vi "luch 2 in 1 - 2v.vi"() -> ()   [LabVIEW 2016]
panel:
  in  "Setup 2":bool
  in  "IBP":bool
  in  "Setup":bool
  in  "Values start":T1=5 items=["External rising edge"=1, "Single shot internal rising edge"=3, "Single shot"=5]
  in  "DZ2K1W":bool
  in  "BZ2K1W":bool
  in  "BZ1K1W":bool
  in  "DZ1K1W":bool
  out "I F0-ethernet 1":string
  in  "F0-ethernet 1":bool
  out "F0-e 3":bool
  out "I: GF":string
  out "GF":bool
  in  "Delay D (0 s)":ext=100.0
  in  "GF":bool
  out "I: FI":string
  out "FI":bool
  in  "Delay C (0 s)":ext=100.0
  in  "FI":bool
  in  "F-R VISAR1":bool
  in  "Delay A (0 s)":ext=100.0
  out "F-R VISAR 1":bool
  out "I: F-R VISAR 1":string
  out "F-R VISAR 2":bool
  out "I: F-R VISAR 2":string
  in  "F-R VISAR2":bool
  in  "Delay B (0 s)":ext=100.0
  in  "WebBrowser":refnum<k7>(container)
  out "Time Stamp":T2
  in  "stop":T3
  out "VISA resource name out":string
  out "I: DZ2K1W":string
  out "DZ2K1W":bool
  out "I: BZ2K1W":string
  out "BZ2K1W":bool
  out "I: BZ1K1W":string
  out "BZ1K1W":bool
  out "I: DZ1K1W":string
  out "DZ1K1W":bool
  out "I: F0-ethernet 5":string
  in  "F0-ethernet 5":bool
  out "F0-e 5":bool
  in  "GF":bool
  in  "FI":bool
  in  "F-R VISAR 4":bool
  in  "F-R VISAR 3":bool
  out "I: BZ1K2W":string
  out "BZ1K2W":bool
  out "I: DZ1K2W":string
  out "DZ1K2W":bool
  out "I: F0-ethernet 4":string
  in  "F0-ethernet 4":bool
  out "F0-e 4":bool
  out "I: BZ2K2W":string
  out "I: DZ2K2W":string
  out "DZ2K2W":bool
  out "BZ2K2W":bool
  in  "BK3":bool
  in  "BK 2":bool
  in  "BK1":bool
  in  "Kamera Y":bool
  out "mod 02":string
  out "mod 01":string
  out "I F0-ethernet 3":string
  in  "F0-ethernet 3":bool
  out "F0-e 1":bool
  out "I: PZS 2 DOP":string
  out "I: PZS 1 DOP":string
  in  "PZS 2 DOP":bool
  in  "PZS 1 DOP":bool
  out "PZS 2 DOP":bool
  out "PZS 1 DOP":bool
  in  "BZ1K2W":bool
  in  "DZ1K2W":bool
  in  "BZ2K2W":bool
  in  "DZ2K2W":bool
  out "I: BK3":string
  out "BK3":bool
  in  "Delay H (0 s)":ext=100.0
  in  "BK3":bool
  in  "Delay G (0 s)":ext=100.0
  in  "BK2":bool
  out "I: BK2":string
  out "BK2":bool
  in  "Delay F (0 s)":ext=100.0
  in  "BK1":bool
  out "I: BK1":string
  out "BK1":bool
  out "I F0-ethernet 2":string
  in  "Delay E (0 s)":ext=100.0
  in  "Kamera Y":bool
  out "I: Kamera Y":string
  out "Kamera Y":bool
  in  "F0-ethernet 2":bool
  out "F0-e 2":bool
  out "error out 2":errorcluster
  out "I 0_3":string
  in  "rele 0_6":bool
  out "modul 03":string
  out "0_3":bool
  out "error out":errorcluster
  # "Ток(A)"
  # "FO-ETHERNET №2"
  # "Гармоника 2"
  # "Ток(A)"
  # "Камеру У"
  # "Камера Б1"
  # "Ток(A)"
  # "Ток(A)"
  # "FO-ETHERNET №4"
  # "1 канал Дальняя Зона"
  # "2 канал Дальняя Зона"
  # "Ток(A)"
  # "Ток(A)"
  # "Задержка E (100~1099ns)"
  # "Задержка F (100~1099ns)"
  # "1 канал Ближняя Зона"
  # "2 канал Ближняя Зона"
  # "Ток(A)"
  # "Ток(A)"
  # "Камера Б2"
  # "Камера Б3"
  # "Ток(A)"
  # "Ток(A)"
  # "Ток(A)"
  # "Гармоника 1"
  # "FO-ETHERNET №5"
  # "1 канал Дальняя Зона"
  # "2 канал Дальняя Зона"
  # "Ток(A)"
  # "Ток(A)"
  # "Ток(A)"
  # "FO-ETHERNET №3"
  # "2 канал Ближняя Зона"
  # "1 канал Ближняя Зона"
  # "Ток (A)"
  # "Ток(A)"
  # "Ток(A)"
  # "ПЗС №1"
  # "Ток(A)"
  # "ПЗС №2"
  # "ИСТОЧНИК БЕСПИРИБОЙНОГО ПИТАНИЯ"
  # "Ток(A)"
  # "FO-ETHERNET №1"
  # "VISAR №2"
  # "VISAR №1"
  # "Ток(A)"
  # "Ток(A)"
  # "Задержка А (100~1099ns)"
  # "Задержка B (100~1099ns)"
  # "Форма имульса"
  # "Глубокий фронт"
  # "Ток(A)"
  # "Ток(A)"
  # "Задержка С (100~1099ns)"
  # "Задержка D (100~1099ns)"
  # "Задержка H (100~1099ns)"
  # "Задержка G (100~1099ns)"
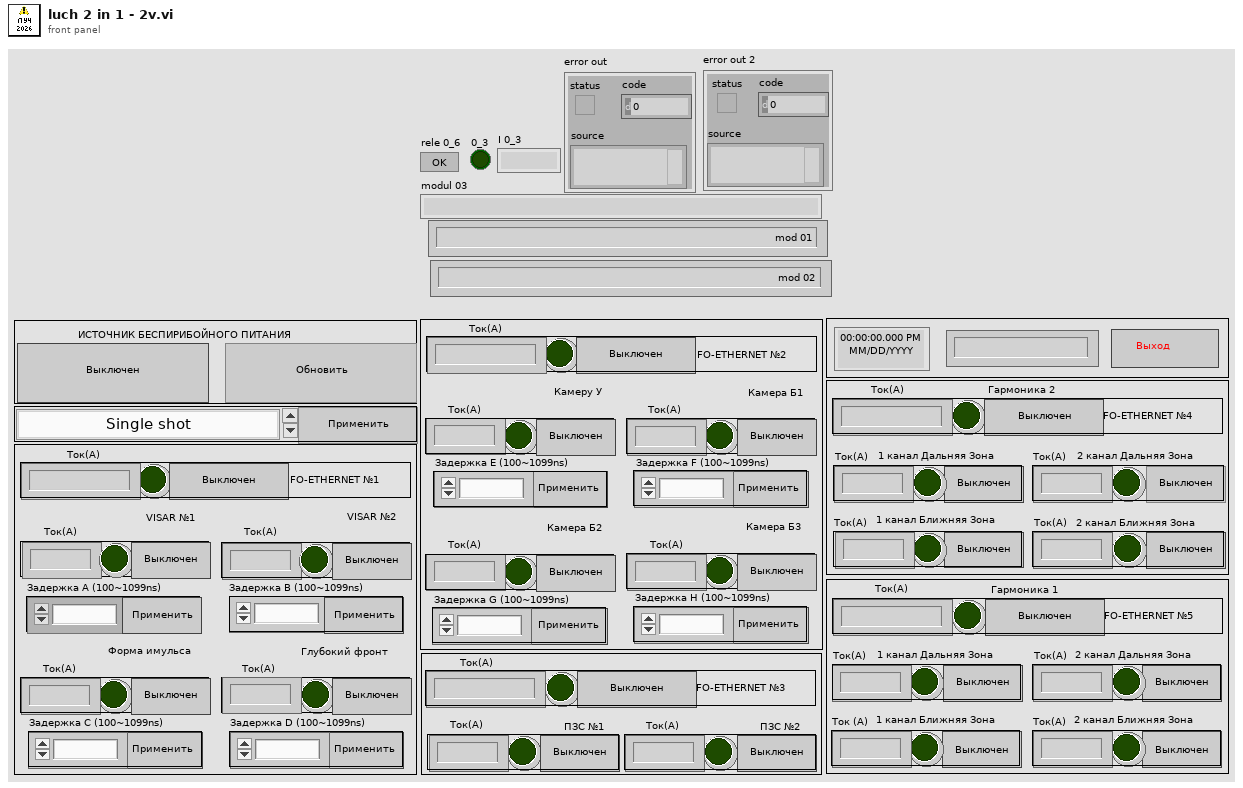
[diagram p1: front panel]
types:
  T1 = typedef "Control 2.ctl" = u16
  T2 = typedef "Control 4.ctl" = timestamp
  T3 = typedef "Control 1.ctl" = bool
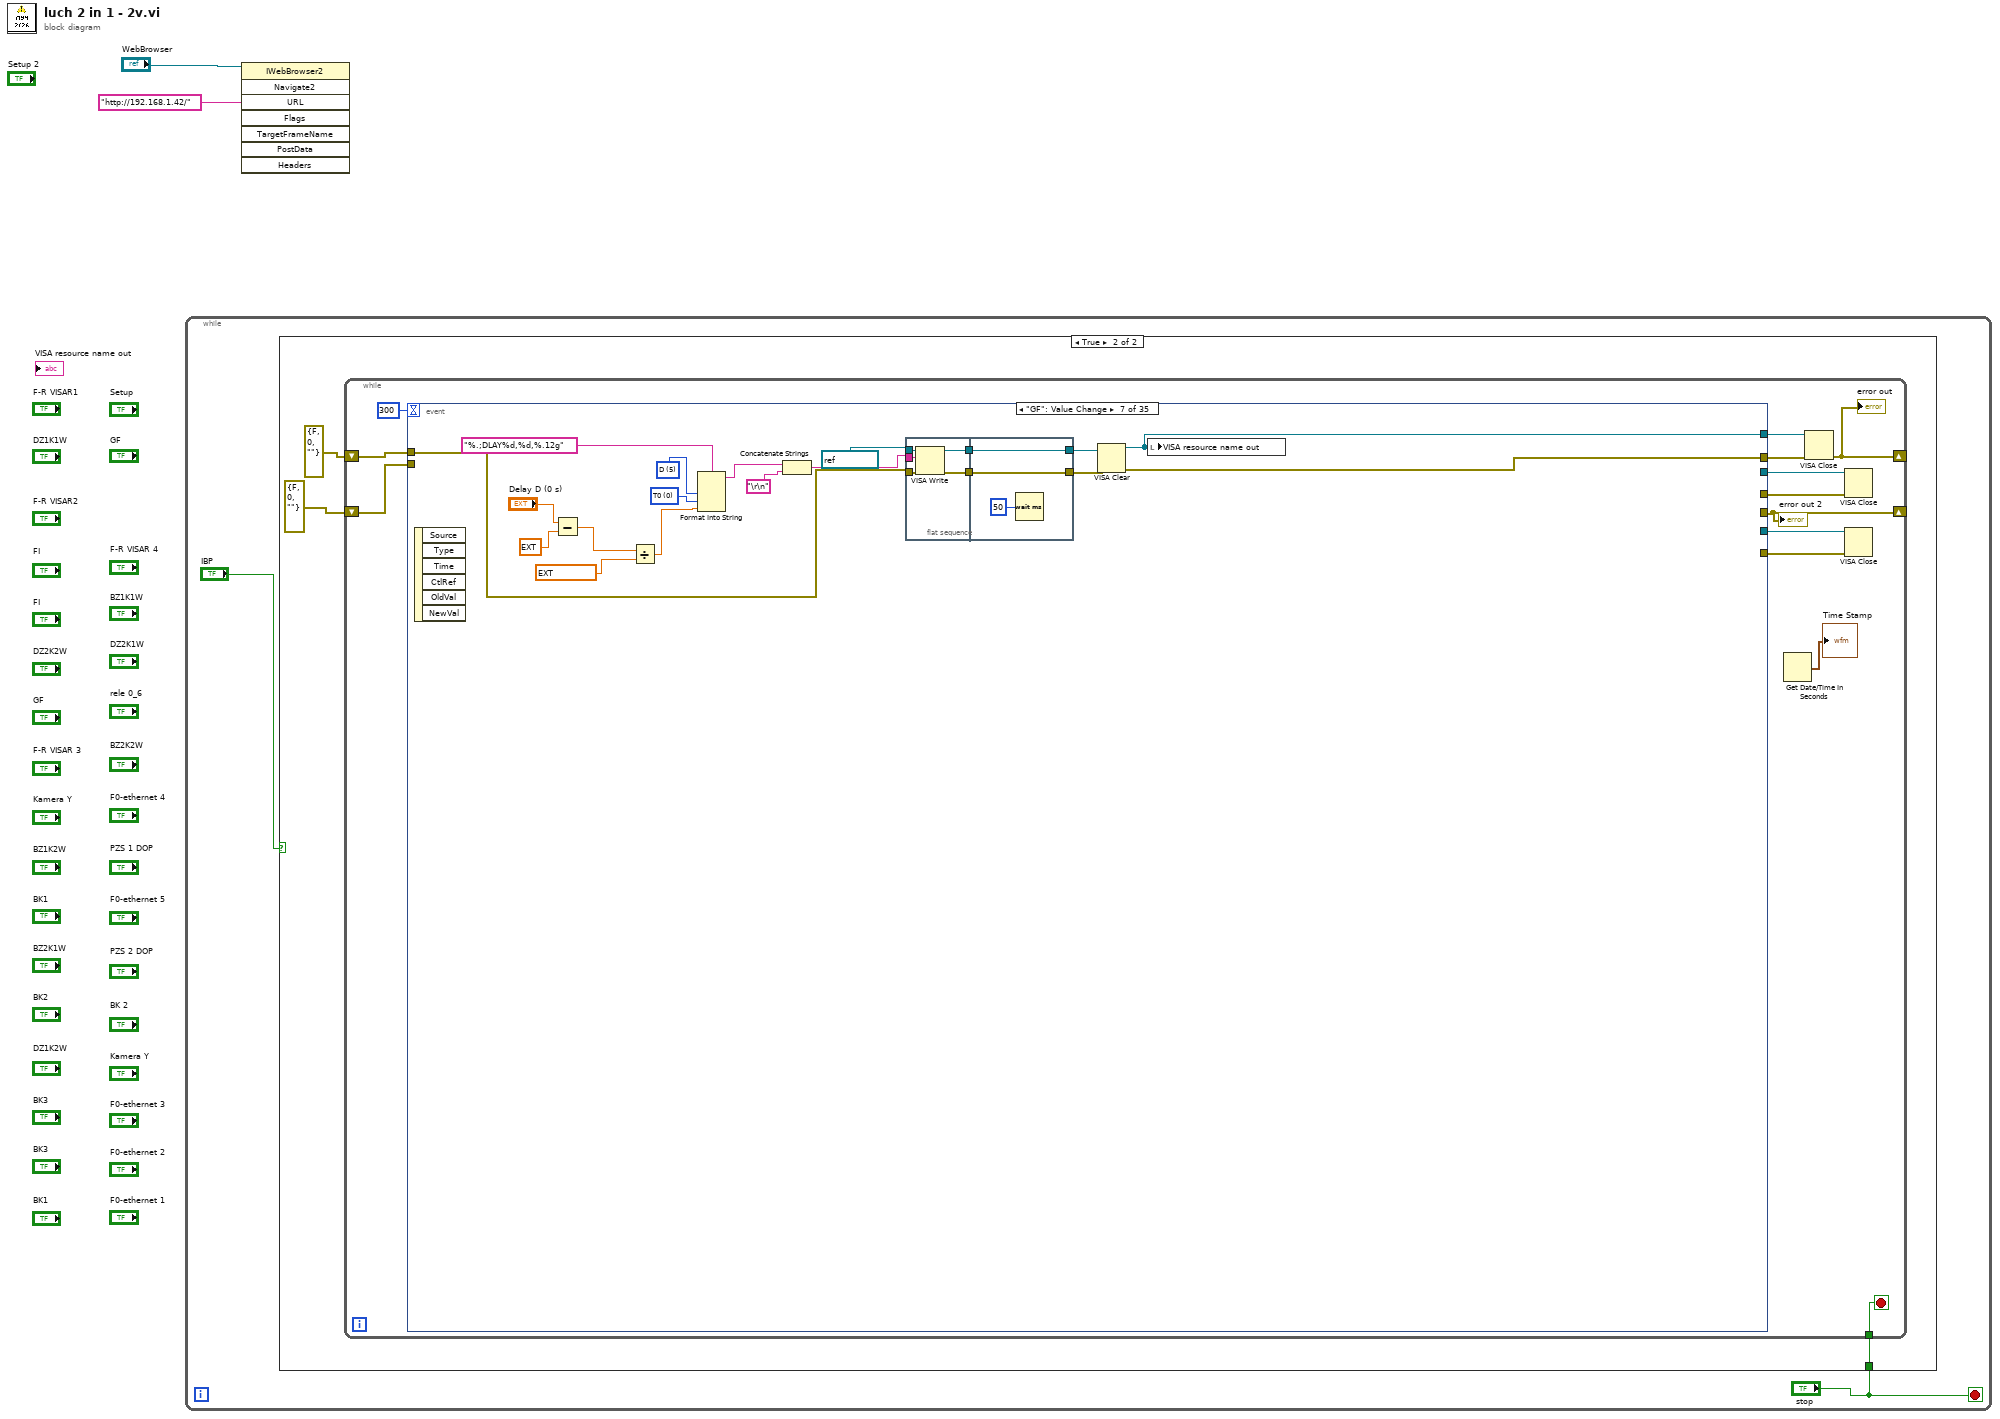
[diagram p0: block diagram]
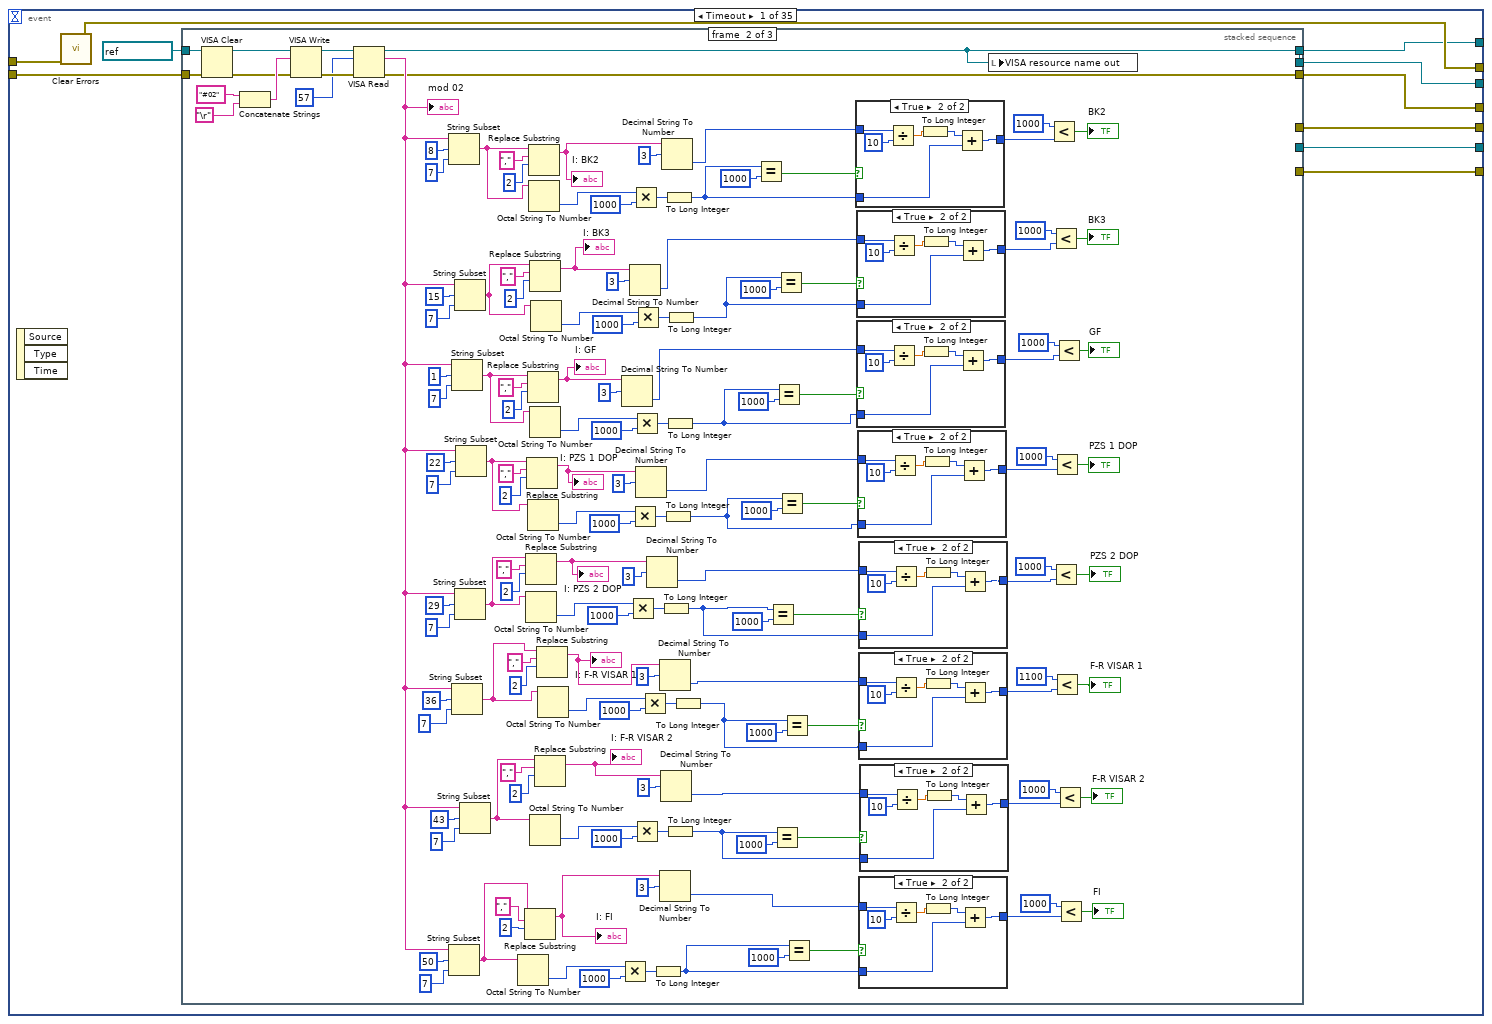
[diagram p3: hidden frame]
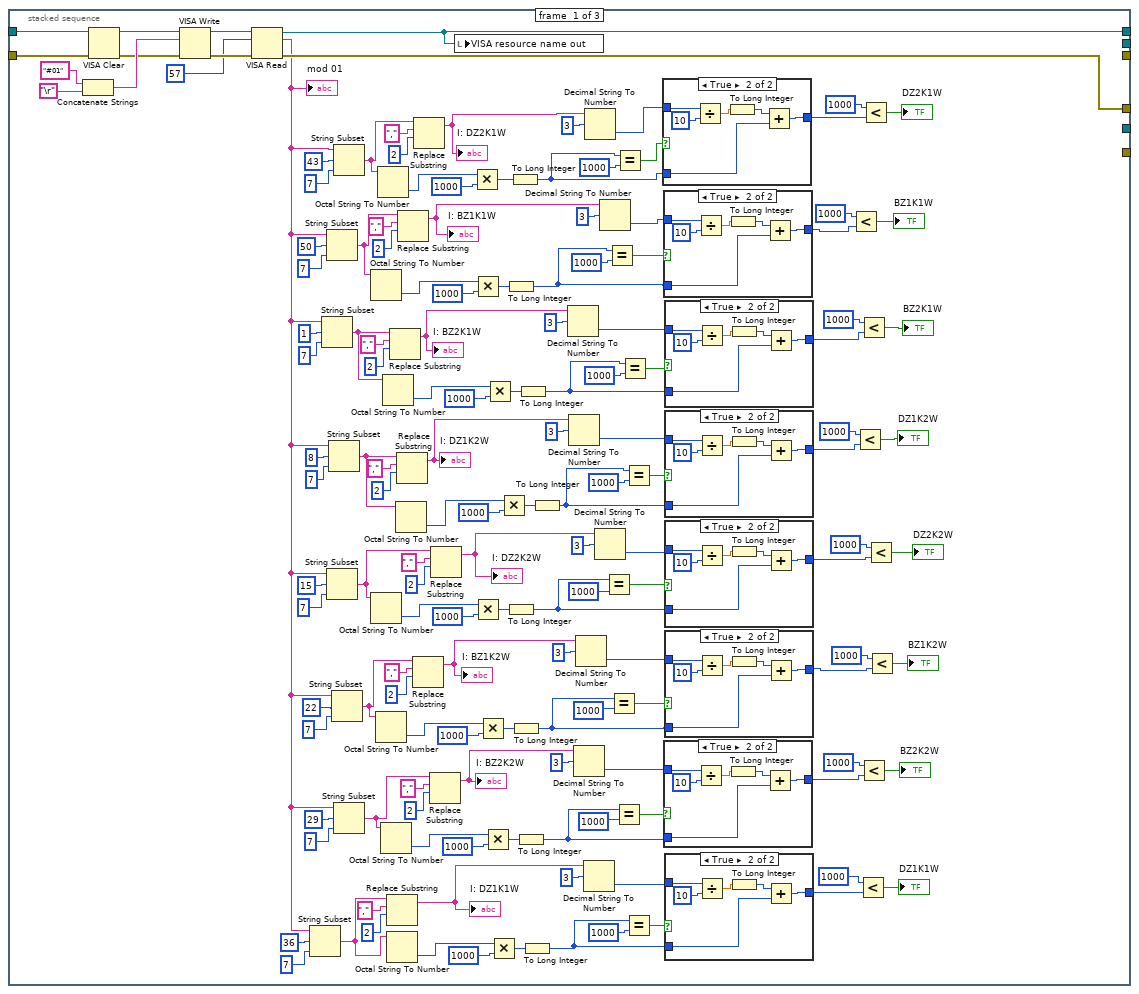
[diagram p4: hidden frame]
diagram:
  n1 = while {
    stop <- "stop" stop-if-true
    n2 = case shown="True" "IBP" {
      tunnel: "stop" -> [_ w5]
      frame False {
      }
      frame True {
        n3 = while {
          shift-right: [w18] -> _
          shift-left: errorcluster {"status"=FALSE, "code"=0, "source"=""} ("error out") -> [w20]
          shift-right: [w11] -> _
          shift-left: errorcluster {"status"=FALSE, "code"=0, "source"=""} ("error out") -> [w19]
          tunnel: w5 -> [w8]
          stop <- w8 stop-if-true
          n4 = event shown="[6] \"GF\": Value Change" {
            selector: _ -> [_ _ _ _ _ _ _ _ _ _ _ _ _ _ _ _ _ _ _ _ _ _ _ _ _ _ _ _ _ _ _ _ _ _ _]
            dyn-events: _ -> [_ _ _ _ _ _ _ _ _ _ _ _ _ _ _ _ _ _ _ _ _ _ _ _ _ _ _ _ _ _ _ _ _ _ _]
            timeout: 300 -> [_ _ _ _ _ _ _ _ _ _ _ _ _ _ _ _ _ _ _ _ _ _ _ _ _ _ _ _ _ _ _ _ _ _ _]
            tunnel: [w29 w647 w650 w720 w747 w775 w801 w828 w854 w882 w909 _ _ _ _ _ _ _ _ _ _ _ _ _ _ _ _ _ _ _ _ _ _ _ _] -> w12
            tunnel: w20 -> [w30 w648 w652 w723 w750 w777 w804 w831 w858 w885 w912 _ _ _ _ _ _ _ _ _ _ _ _ _ _ _ _ _ _ _ _ _ _ _ _]
            tunnel: w19 -> [w27 w644 _ _ _ _ _ _ _ _ _ w934 w962 w995 w1026 w1057 w1088 w1119 w1150 w1181 w1213 w1243 w1274 w1305 w1336 w1367 w1399 w1429 w1460 w1491 w1522 w1553 w1584 w1615 w1646]
            tunnel: [w26 w643 _ _ _ _ _ _ _ _ _ w930 w961 w992 w1023 w1055 w1085 w1117 w1147 w1178 w1209 w1240 w1271 w1302 w1333 w1364 w1395 w1426 w1457 w1488 w1519 w1550 w1581 w1612 w1643] -> w11
            tunnel: [w25 _ w649 w716 w743 w770 w797 w824 w851 w878 w905 w927 w958 w989 w1020 w1051 w1082 w1113 w1144 w1175 w1206 w1237 w1268 w1299 w1330 w1361 w1392 w1423 w1454 w1485 w1516 w1547 w1578 w1609 w1640] -> w17
            tunnel: [w24 _ _ _ _ _ _ _ _ _ _ _ _ _ _ _ _ _ _ _ _ _ _ _ _ _ _ _ _ _ _ _ _ _ _] -> w16
            tunnel: [w23 _ _ _ _ _ _ _ _ _ _ _ _ _ _ _ _ _ _ _ _ _ _ _ _ _ _ _ _ _ _ _ _ _ _] -> w15
            tunnel: [w22 _ _ _ _ _ _ _ _ _ _ _ _ _ _ _ _ _ _ _ _ _ _ _ _ _ _ _ _ _ _ _ _ _ _] -> w14
            tunnel: [w21 _ _ _ _ _ _ _ _ _ _ _ _ _ _ _ _ _ _ _ _ _ _ _ _ _ _ _ _ _ _ _ _ _ _] -> w13
            event Timeout {
              n5 = event-data() -> ()  [unwired: 1 in, 3 out]
              n6 = call <vilib>:"Clear Errors.vi"("error in (no error)"=w30) -> ("error out"=w29:errorcluster)  [unwired: 5 in, 1 out]
              n7 = stacked-sequence {
                tunnel: refnum<visa-resource-name> "Adam" ("VISA resource name") -> [w107 w311 w535]
                tunnel: [w141 _ _] -> w26
                tunnel: w27 -> [w106 w313 w532]
                tunnel: [w103 _ _] -> w25
                tunnel: [_ w309 _] -> w24
                tunnel: [_ w308 _] -> w23
                tunnel: [_ _ w515] -> w22
                tunnel: [_ _ w514] -> w21
                frame #0 {
                  n8 = Concatenate Strings("#01" ("string"), "\r") -> (w179:string)
                  n9 = VISA Clear(VISA resource name=w107, error in (no error)=w106) -> (VISA resource name out=w104:refnum<visa-resource-name>, error out=w105:errorcluster)
                  n10 = VISA Write(VISA resource name=w104, write buffer=w179, error in (no error)=w105) -> (VISA resource name out=w144:refnum<visa-resource-name>, error out=w143:errorcluster)  [unwired: 1 out]
                  n11 = VISA Read(VISA resource name=w144, byte count=u32 57, error in (no error)=w143) -> (VISA resource name out=w103:refnum<visa-resource-name>, read buffer=w124:string, error out=w141:errorcluster)  [unwired: 1 out]
                  "mod 01" <- w124
                  n12 = String Subset(string=w124, offset (0)=36, length (rest)=7 ("length (rest)")) -> (substring=w98:string)
                  n13 = String Subset(string=w124, offset (0)=1, length (rest)=7 ("length (rest)")) -> (substring=w53:string)
                  n14 = String Subset(string=w124, offset (0)=50, length (rest)=7 ("length (rest)")) -> (substring=w43:string)
                  n15 = String Subset(string=w124, offset (0)=15, length (rest)=7 ("length (rest)")) -> (substring=w71:string)
                  n16 = String Subset(string=w124, offset (0)=8, length (rest)=7 ("length (rest)")) -> (substring=w58:string)
                  n17 = String Subset(string=w124, offset (0)=22, length (rest)=7 ("length (rest)")) -> (substring=w76:string)
                  n18 = String Subset(string=w124, offset (0)=43, length (rest)=7 ("length (rest)")) -> (substring=w34:string)
                  n19 = String Subset(string=w124, offset (0)=29, length (rest)=7 ("length (rest)")) -> (substring=w88:string)
                  n20 = Octal String To Number(4:w43) -> (0:w47:u32)  [unwired: 2 in, 1 out]
                  n21 = Octal String To Number(4:w71) -> (0:w75:u32)  [unwired: 2 in, 1 out]
                  n22 = Octal String To Number(4:w76) -> (0:w82:u32)  [unwired: 2 in, 1 out]
                  n23 = Octal String To Number(4:w34) -> (0:w38:u32)  [unwired: 2 in, 1 out]
                  n24 = Octal String To Number(4:w88) -> (0:w91:u32)  [unwired: 2 in, 1 out]
                  n25 = Octal String To Number(4:w53) -> (0:w57:u32)  [unwired: 2 in, 1 out]
                  n26 = Replace Substring(3:2 ("offset (0)"), 4:"," ("substring (\"\")"), 5:w98) -> (1:w112:string)  [unwired: 1 in, 1 out]
                  "I: DZ1K1W" <- w112
                  n27 = Octal String To Number(4:w98) -> (0:w102:u32)  [unwired: 2 in, 1 out]
                  n28 = Replace Substring(3:2 ("offset (0)"), 4:"," ("substring (\"\")"), 5:w53) -> (1:w123:string)  [unwired: 1 in, 1 out]
                  "I: BZ2K1W" <- w123
                  n29 = Octal String To Number(4:w58) -> (0:w66:u32)  [unwired: 2 in, 1 out]
                  n30 = Replace Substring(3:2 ("offset (0)"), 4:"," ("substring (\"\")"), 5:w58) -> (1:w121:string)  [unwired: 1 in, 1 out]
                  "I: DZ1K2W" <- w121
                  n31 = Replace Substring(3:2 ("offset (0)"), 4:"," ("substring (\"\")"), 5:w43) -> (1:w109:string)  [unwired: 1 in, 1 out]
                  "I: BZ1K1W" <- w109
                  n32 = Replace Substring(3:2 ("offset (0)"), 4:"," ("substring (\"\")"), 5:w76) -> (1:w117:string)  [unwired: 1 in, 1 out]
                  "I: BZ1K2W" <- w117
                  n33 = Replace Substring(3:2 ("offset (0)"), 4:"," ("substring (\"\")"), 5:w34) -> (1:w110:string)  [unwired: 1 in, 1 out]
                  "I: DZ2K1W" <- w110
                  n34 = Replace Substring(3:2 ("offset (0)"), 4:"," ("substring (\"\")"), 5:w88) -> (1:w115:string)  [unwired: 1 in, 1 out]
                  "I: BZ2K2W" <- w115
                  n35 = Replace Substring(3:2 ("offset (0)"), 4:"," ("substring (\"\")"), 5:w71) -> (1:w119:string)  [unwired: 1 in, 1 out]
                  "I: DZ2K2W" <- w119
                  n36 = local write "VISA resource name out"(w103) -> ()
                  n37 = Multiply(x=w38, y=u32 1000) -> (x*y=w36:u32)
                  n38 = Multiply(x=w47, y=u32 1000) -> (x*y=w45:u32)
                  n39 = Multiply(x=w75, y=u32 1000) -> (x*y=w73:u32)
                  n40 = Multiply(x=w82, y=u32 1000) -> (x*y=w80:u32)
                  n41 = Multiply(x=w91, y=u32 1000) -> (x*y=w89:u32)
                  n42 = Multiply(x=w57, y=u32 1000) -> (x*y=w55:u32)
                  n43 = Multiply(x=w102, y=u32 1000) -> (x*y=w100:u32)
                  n44 = Multiply(x=w66, y=u32 1000) -> (x*y=w64:u32)
                  n45 = To Long Integer(number=w45) -> (32bit integer=w42:i32)
                  n46 = To Long Integer(number=w73) -> (32bit integer=w70:i32)
                  n47 = To Long Integer(number=w36) -> (32bit integer=w33:i32)
                  n48 = To Long Integer(number=w80) -> (32bit integer=w78:i32)
                  n49 = To Long Integer(number=w89) -> (32bit integer=w85:i32)
                  n50 = To Long Integer(number=w55) -> (32bit integer=w52:i32)
                  n51 = To Long Integer(number=w100) -> (32bit integer=w96:i32)
                  n52 = To Long Integer(number=w64) -> (32bit integer=w61:i32)
                  n53 = Decimal String To Number(string=w123, offset=3) -> (number=w49:i32)  [unwired: 1 in, 1 out]
                  n54 = Decimal String To Number(string=w121, offset=3) -> (number=w59:i32)  [unwired: 1 in, 1 out]
                  n55 = Decimal String To Number(string=w115, offset=3) -> (number=w92:i32)  [unwired: 1 in, 1 out]
                  n56 = Decimal String To Number(string=w117, offset=3) -> (number=w83:i32)  [unwired: 1 in, 1 out]
                  n57 = Decimal String To Number(string=w112, offset=3) -> (number=w95:i32)  [unwired: 1 in, 1 out]
                  n58 = Decimal String To Number(string=w110, offset=3) -> (number=w31:i32)  [unwired: 1 in, 1 out]
                  n59 = Decimal String To Number(string=w119, offset=3) -> (number=w67:i32)  [unwired: 1 in, 1 out]
                  n60 = Decimal String To Number(string=w109, offset=3) -> (number=w40:i32)  [unwired: 1 in, 1 out]
                  n61 = Equal?(x=w70, y=1000) -> (x = y?=w69:bool)
                  n62 = Equal?(x=w42, y=1000) -> (x = y?=w41:bool)
                  n63 = Equal?(x=w78, y=1000) -> (x = y?=w77:bool)
                  n64 = Equal?(x=w85, y=1000) -> (x = y?=w86:bool)
                  n65 = Equal?(x=w33, y=1000) -> (x = y?=w32:bool)
                  n66 = Equal?(x=w52, y=1000) -> (x = y?=w51:bool)
                  n67 = Equal?(x=w61, y=1000) -> (x = y?=w62:bool)
                  n68 = Equal?(x=w96, y=1000) -> (x = y?=w97:bool)
                  n69 = case shown="True" w32 {
                    tunnel: w31 -> [w180 w186]
                    tunnel: w33 -> [_ w184]
                    tunnel: [w180 w183] -> w39
                    frame False {
                    }
                    frame True {
                      n70 = Divide(x=w186, y=10) -> (x/y=w182:dbl)
                      n71 = To Long Integer(number=w182) -> (32bit integer=w181:i32)
                      n72 = Add(x=w181, y=w184) -> (x+y=w183:i32)
                    }
                  }
                  n73 = case shown="True" w41 {
                    tunnel: w40 -> [w187 w193]
                    tunnel: w42 -> [_ w191]
                    tunnel: [w187 w190] -> w48
                    frame False {
                    }
                    frame True {
                      n74 = Divide(x=w193, y=10) -> (x/y=w189:dbl)
                      n75 = To Long Integer(number=w189) -> (32bit integer=w188:i32)
                      n76 = Add(x=w188, y=w191) -> (x+y=w190:i32)
                    }
                  }
                  n77 = case shown="True" w86 {
                    tunnel: w92 -> [w222 w228]
                    tunnel: w85 -> [_ w226]
                    tunnel: [w222 w225] -> w93
                    frame False {
                    }
                    frame True {
                      n78 = Divide(x=w228, y=10) -> (x/y=w224:dbl)
                      n79 = To Long Integer(number=w224) -> (32bit integer=w223:i32)
                      n80 = Add(x=w223, y=w226) -> (x+y=w225:i32)
                    }
                  }
                  n81 = case shown="True" w51 {
                    tunnel: w49 -> [w194 w200]
                    tunnel: w52 -> [_ w198]
                    tunnel: [w194 w197] -> w50
                    frame False {
                    }
                    frame True {
                      n82 = Divide(x=w200, y=10) -> (x/y=w196:dbl)
                      n83 = To Long Integer(number=w196) -> (32bit integer=w195:i32)
                      n84 = Add(x=w195, y=w198) -> (x+y=w197:i32)
                    }
                  }
                  n85 = case shown="True" w62 {
                    tunnel: w59 -> [w201 w207]
                    tunnel: w61 -> [_ w205]
                    tunnel: [w201 w204] -> w60
                    frame False {
                    }
                    frame True {
                      n86 = Divide(x=w207, y=10) -> (x/y=w203:dbl)
                      n87 = To Long Integer(number=w203) -> (32bit integer=w202:i32)
                      n88 = Add(x=w202, y=w205) -> (x+y=w204:i32)
                    }
                  }
                  n89 = case shown="True" w69 {
                    tunnel: w67 -> [w208 w214]
                    tunnel: w70 -> [_ w212]
                    tunnel: [w208 w211] -> w68
                    frame False {
                    }
                    frame True {
                      n90 = Divide(x=w214, y=10) -> (x/y=w210:dbl)
                      n91 = To Long Integer(number=w210) -> (32bit integer=w209:i32)
                      n92 = Add(x=w209, y=w212) -> (x+y=w211:i32)
                    }
                  }
                  n93 = case shown="True" w77 {
                    tunnel: w83 -> [w215 w221]
                    tunnel: w78 -> [_ w219]
                    tunnel: [w215 w218] -> w84
                    frame False {
                    }
                    frame True {
                      n94 = Divide(x=w221, y=10) -> (x/y=w217:dbl)
                      n95 = To Long Integer(number=w217) -> (32bit integer=w216:i32)
                      n96 = Add(x=w216, y=w219) -> (x+y=w218:i32)
                    }
                  }
                  n97 = case shown="True" w97 {
                    tunnel: w95 -> [w229 w235]
                    tunnel: w96 -> [_ w233]
                    tunnel: [w229 w232] -> w94
                    frame False {
                    }
                    frame True {
                      n98 = Divide(x=w235, y=10) -> (x/y=w231:dbl)
                      n99 = To Long Integer(number=w231) -> (32bit integer=w230:i32)
                      n100 = Add(x=w230, y=w233) -> (x+y=w232:i32)
                    }
                  }
                  n101 = Less?(x=1000, y=w48) -> (x < y?=→"BZ1K1W":bool)
                  n102 = Less?(x=1000, y=w60) -> (x < y?=→"DZ1K2W":bool)
                  n103 = Less?(x=1000, y=w94) -> (x < y?=→"DZ1K1W":bool)
                  n104 = Less?(x=1000, y=w50) -> (x < y?=→"BZ2K1W":bool)
                  n105 = Less?(x=1000, y=w93) -> (x < y?=→"BZ2K2W":bool)
                  n106 = Less?(x=1000, y=w39) -> (x < y?=→"DZ2K1W":bool)
                  n107 = Less?(x=1000, y=w68) -> (x < y?=→"DZ2K2W":bool)
                  n108 = Less?(x=1000, y=w84) -> (x < y?=→"BZ1K2W":bool)
                }
                frame #1 {
                  n109 = VISA Clear(VISA resource name=w311, error in (no error)=w313) -> (VISA resource name out=w310:refnum<visa-resource-name>, error out=w312:errorcluster)
                  n110 = Concatenate Strings("#02" ("string"), "\r") -> (w384:string)
                  n111 = VISA Write(VISA resource name=w310, write buffer=w384, error in (no error)=w312) -> (VISA resource name out=w349:refnum<visa-resource-name>, error out=w348:errorcluster)  [unwired: 1 out]
                  n112 = VISA Read(VISA resource name=w349, byte count=u32 57, error in (no error)=w348) -> (VISA resource name out=w309:refnum<visa-resource-name>, read buffer=w330:string, error out=w308:errorcluster)  [unwired: 1 out]
                  "mod 02" <- w330
                  n113 = String Subset(string=w330, offset (0)=8, length (rest)=7 ("length (rest)")) -> (substring=w240:string)
                  n114 = String Subset(string=w330, offset (0)=50, length (rest)=7 ("length (rest)")) -> (substring=w307:string)
                  n115 = String Subset(string=w330, offset (0)=1, length (rest)=7 ("length (rest)")) -> (substring=w258:string)
                  n116 = String Subset(string=w330, offset (0)=36, length (rest)=7 ("length (rest)")) -> (substring=w285:string)
                  n117 = String Subset(string=w330, offset (0)=15, length (rest)=7 ("length (rest)")) -> (substring=w246:string)
                  n118 = String Subset(string=w330, offset (0)=29, length (rest)=7 ("length (rest)")) -> (substring=w277:string)
                  n119 = String Subset(string=w330, offset (0)=22, length (rest)=7 ("length (rest)")) -> (substring=w267:string)
                  n120 = String Subset(string=w330, offset (0)=43, length (rest)=7 ("length (rest)")) -> (substring=w294:string)
                  n121 = Octal String To Number(4:w307) -> (0:w306:u32)  [unwired: 2 in, 1 out]
                  n122 = Replace Substring(3:2 ("offset (0)"), 4:"," ("substring (\"\")"), 5:w307) -> (1:w316:string)  [unwired: 1 in, 1 out]
                  "I: FI" <- w316
                  n123 = Replace Substring(3:2 ("offset (0)"), 4:"," ("substring (\"\")"), 5:w277) -> (1:w320:string)  [unwired: 1 in, 1 out]
                  "I: PZS 2 DOP" <- w320
                  n124 = Octal String To Number(4:w277) -> (0:w281:u32)  [unwired: 2 in, 1 out]
                  n125 = Replace Substring(3:2 ("offset (0)"), 4:"," ("substring (\"\")"), 5:w267) -> (1:w323:string)  [unwired: 1 in, 1 out]
                  "I: PZS 1 DOP" <- w323
                  n126 = Replace Substring(3:2 ("offset (0)"), 4:"," ("substring (\"\")"), 5:w258) -> (1:w328:string)  [unwired: 1 in, 1 out]
                  "I: GF" <- w328
                  n127 = Octal String To Number(4:w267) -> (0:w271:u32)  [unwired: 2 in, 1 out]
                  n128 = Replace Substring(3:2 ("offset (0)"), 4:"," ("substring (\"\")"), 5:w240) -> (1:w326:string)  [unwired: 1 in, 1 out]
                  "I: BK2" <- w326
                  n129 = Octal String To Number(4:w240) -> (0:w244:u32)  [unwired: 2 in, 1 out]
                  n130 = Replace Substring(3:2 ("offset (0)"), 4:"," ("substring (\"\")"), 5:w246) -> (1:w325:string)  [unwired: 1 in, 1 out]
                  "I: BK3" <- w325
                  n131 = Octal String To Number(4:w258) -> (0:w262:u32)  [unwired: 2 in, 1 out]
                  n132 = Octal String To Number(4:w294) -> (0:w298:u32)  [unwired: 2 in, 1 out]
                  n133 = Octal String To Number(4:w246) -> (0:w252:u32)  [unwired: 2 in, 1 out]
                  n134 = Replace Substring(3:2 ("offset (0)"), 4:"," ("substring (\"\")"), 5:w294) -> (1:w317:string)  [unwired: 1 in, 1 out]
                  "I: F-R VISAR 2" <- w317
                  n135 = Replace Substring(3:2 ("offset (0)"), 4:"," ("substring (\"\")"), 5:w285) -> (1:w318:string)  [unwired: 1 in, 1 out]
                  "I: F-R VISAR 1" <- w318
                  n136 = Octal String To Number(4:w285) -> (0:w289:u32)  [unwired: 2 in, 1 out]
                  n137 = Multiply(x=w306, y=u32 1000) -> (x*y=w304:u32)
                  n138 = Decimal String To Number(string=w328, offset=3) -> (number=w255:i32)  [unwired: 1 in, 1 out]
                  n139 = Multiply(x=w281, y=u32 1000) -> (x*y=w279:u32)
                  n140 = Decimal String To Number(string=w325, offset=3) -> (number=w245:i32)  [unwired: 1 in, 1 out]
                  n141 = Multiply(x=w271, y=u32 1000) -> (x*y=w269:u32)
                  n142 = Multiply(x=w244, y=u32 1000) -> (x*y=w242:u32)
                  n143 = Multiply(x=w262, y=u32 1000) -> (x*y=w260:u32)
                  n144 = Multiply(x=w298, y=u32 1000) -> (x*y=w296:u32)
                  n145 = Multiply(x=w252, y=u32 1000) -> (x*y=w250:u32)
                  n146 = Decimal String To Number(string=w323, offset=3) -> (number=w263:i32)  [unwired: 1 in, 1 out]
                  n147 = Multiply(x=w289, y=u32 1000) -> (x*y=w287:u32)
                  n148 = Decimal String To Number(string=w320, offset=3) -> (number=w275:i32)  [unwired: 1 in, 1 out]
                  n149 = To Long Integer(number=w304) -> (32bit integer=w300:i32)
                  n150 = Decimal String To Number(string=w318, offset=3) -> (number=w282:i32)  [unwired: 1 in, 1 out]
                  n151 = Decimal String To Number(string=w316, offset=3) -> (number=w301:i32)  [unwired: 1 in, 1 out]
                  n152 = To Long Integer(number=w279) -> (32bit integer=w272:i32)
                  n153 = Decimal String To Number(string=w317, offset=3) -> (number=w291:i32)  [unwired: 1 in, 1 out]
                  n154 = Decimal String To Number(string=w326, offset=3) -> (number=w236:i32)  [unwired: 1 in, 1 out]
                  n155 = To Long Integer(number=w269) -> (32bit integer=w264:i32)
                  n156 = To Long Integer(number=w242) -> (32bit integer=w237:i32)
                  n157 = To Long Integer(number=w260) -> (32bit integer=w256:i32)
                  n158 = To Long Integer(number=w296) -> (32bit integer=w292:i32)
                  n159 = To Long Integer(number=w250) -> (32bit integer=w247:i32)
                  n160 = To Long Integer(number=w287) -> (32bit integer=w283:i32)
                  n161 = Equal?(x=w237, y=1000) -> (x = y?=w238:bool)
                  n162 = Equal?(x=w272, y=1000) -> (x = y?=w276:bool)
                  n163 = Equal?(x=w292, y=1000) -> (x = y?=w293:bool)
                  n164 = Equal?(x=w256, y=1000) -> (x = y?=w257:bool)
                  n165 = Equal?(x=w247, y=1000) -> (x = y?=w248:bool)
                  n166 = Equal?(x=w264, y=1000) -> (x = y?=w265:bool)
                  n167 = Equal?(x=w283, y=1000) -> (x = y?=w284:bool)
                  n168 = Equal?(x=w300, y=1000) -> (x = y?=w302:bool)
                  n169 = case shown="True" w238 {
                    tunnel: w236 -> [w385 w391]
                    tunnel: w237 -> [_ w389]
                    tunnel: [w385 w388] -> w239
                    frame False {
                    }
                    frame True {
                      n170 = Divide(x=w391, y=10) -> (x/y=w387:dbl)
                      n171 = To Long Integer(number=w387) -> (32bit integer=w386:i32)
                      n172 = Add(x=w386, y=w389) -> (x+y=w388:i32)
                    }
                  }
                  n173 = case shown="True" w248 {
                    tunnel: w245 -> [w392 w398]
                    tunnel: w247 -> [_ w396]
                    tunnel: [w392 w395] -> w253
                    frame False {
                    }
                    frame True {
                      n174 = Divide(x=w398, y=10) -> (x/y=w394:dbl)
                      n175 = To Long Integer(number=w394) -> (32bit integer=w393:i32)
                      n176 = Add(x=w393, y=w396) -> (x+y=w395:i32)
                    }
                  }
                  n177 = case shown="True" w257 {
                    tunnel: w255 -> [w399 w405]
                    tunnel: w256 -> [_ w403]
                    tunnel: [w399 w402] -> w254
                    frame False {
                    }
                    frame True {
                      n178 = Divide(x=w405, y=10) -> (x/y=w401:dbl)
                      n179 = To Long Integer(number=w401) -> (32bit integer=w400:i32)
                      n180 = Add(x=w400, y=w403) -> (x+y=w402:i32)
                    }
                  }
                  n181 = case shown="True" w265 {
                    tunnel: w263 -> [w406 w412]
                    tunnel: w264 -> [_ w410]
                    tunnel: [w406 w409] -> w266
                    frame False {
                    }
                    frame True {
                      n182 = Divide(x=w412, y=10) -> (x/y=w408:dbl)
                      n183 = To Long Integer(number=w408) -> (32bit integer=w407:i32)
                      n184 = Add(x=w407, y=w410) -> (x+y=w409:i32)
                    }
                  }
                  n185 = case shown="True" w276 {
                    tunnel: w275 -> [w413 w419]
                    tunnel: w272 -> [_ w417]
                    tunnel: [w413 w416] -> w273
                    frame False {
                    }
                    frame True {
                      n186 = Divide(x=w419, y=10) -> (x/y=w415:dbl)
                      n187 = To Long Integer(number=w415) -> (32bit integer=w414:i32)
                      n188 = Add(x=w414, y=w417) -> (x+y=w416:i32)
                    }
                  }
                  n189 = case shown="True" w284 {
                    tunnel: w282 -> [w420 w426]
                    tunnel: w283 -> [_ w424]
                    tunnel: [w420 w423] -> w274
                    frame False {
                    }
                    frame True {
                      n190 = Divide(x=w426, y=10) -> (x/y=w422:dbl)
                      n191 = To Long Integer(number=w422) -> (32bit integer=w421:i32)
                      n192 = Add(x=w421, y=w424) -> (x+y=w423:i32)
                    }
                  }
                  n193 = case shown="True" w302 {
                    tunnel: w301 -> [w434 w440]
                    tunnel: w300 -> [_ w438]
                    tunnel: [w434 w437] -> w299
                    frame False {
                    }
                    frame True {
                      n194 = Divide(x=w440, y=10) -> (x/y=w436:dbl)
                      n195 = To Long Integer(number=w436) -> (32bit integer=w435:i32)
                      n196 = Add(x=w435, y=w438) -> (x+y=w437:i32)
                    }
                  }
                  n197 = case shown="True" w293 {
                    tunnel: w291 -> [w427 w433]
                    tunnel: w292 -> [_ w431]
                    tunnel: [w427 w430] -> w290
                    frame False {
                    }
                    frame True {
                      n198 = Divide(x=w433, y=10) -> (x/y=w429:dbl)
                      n199 = To Long Integer(number=w429) -> (32bit integer=w428:i32)
                      n200 = Add(x=w428, y=w431) -> (x+y=w430:i32)
                    }
                  }
                  n201 = local write "VISA resource name out"(w309) -> ()
                  n202 = Less?(x=1000, y=w239) -> (x < y?=→"BK2":bool)
                  n203 = Less?(x=1000, y=w253) -> (x < y?=→"BK3":bool)
                  n204 = Less?(x=1000, y=w273) -> (x < y?=→"PZS 2 DOP":bool)
                  n205 = Less?(x=1000, y=w266) -> (x < y?=→"PZS 1 DOP":bool)
                  n206 = Less?(x=1100, y=w274) -> (x < y?=→"F-R VISAR 1":bool)
                  n207 = Less?(x=1000, y=w254) -> (x < y?=→"GF":bool)
                  n208 = Less?(x=1000, y=w290) -> (x < y?=→"F-R VISAR 2":bool)
                  n209 = Less?(x=1000, y=w299) -> (x < y?=→"FI":bool)
                }
                frame #2 {
                  w531 = "" ("string")
                  n210 = VISA Clear(VISA resource name=w535, error in (no error)=w532) -> (VISA resource name out=w533:refnum<visa-resource-name>, error out=w534:errorcluster)
                  n211 = Concatenate Strings("#03" ("string"), "\r") -> (w586:string)
                  n212 = VISA Write(VISA resource name=w533, write buffer=w586, error in (no error)=w534) -> (VISA resource name out=w514:refnum<visa-resource-name>, error out=w515:errorcluster)  [unwired: 1 out]
                  n213 = String Subset(string=w531, offset (0)=29, length (rest)=7 ("length (rest)")) -> (substring=w470:string)
                  n214 = String Subset(string=w531, offset (0)=8, length (rest)=7 ("length (rest)")) -> (substring=w443:string)
                  n215 = String Subset(string=w531, offset (0)=1, length (rest)=7 ("length (rest)")) -> (substring=w481:string)
                  n216 = String Subset(string=w531, offset (0)=36, length (rest)=7 ("length (rest)")) -> (substring=w487:string)
                  n217 = String Subset(string=w531, offset (0)=43, length (rest)=7 ("length (rest)")) -> (substring=w497:string)
                  n218 = String Subset(string=w531, offset (0)=50, length (rest)=7 ("length (rest)")) -> (substring=w504:string)
                  n219 = String Subset(string=w531, offset (0)=22, length (rest)=7 ("length (rest)")) -> (substring=w461:string)
                  n220 = String Subset(string=w531, offset (0)=15, length (rest)=7 ("length (rest)")) -> (substring=w454:string)
                  n221 = Octal String To Number(4:w461) -> (0:w462:u32)  [unwired: 2 in, 1 out]
                  n222 = Octal String To Number(4:w504) -> (0:w510:u32)  [unwired: 2 in, 1 out]
                  n223 = Octal String To Number(4:w443) -> (0:w447:u32)  [unwired: 2 in, 1 out]
                  n224 = Octal String To Number(4:w481) -> (0:w485:u32)  [unwired: 2 in, 1 out]
                  n225 = Octal String To Number(4:w487) -> (0:w493:u32)  [unwired: 2 in, 1 out]
                  n226 = Octal String To Number(4:w470) -> (0:w471:u32)  [unwired: 2 in, 1 out]
                  n227 = Octal String To Number(4:w497) -> (0:w501:u32)  [unwired: 2 in, 1 out]
                  n228 = Octal String To Number(4:w454) -> (0:w458:u32)  [unwired: 2 in, 1 out]
                  n229 = Replace Substring(3:2 ("offset (0)"), 4:"," ("substring (\"\")"), 5:w443) -> (1:w528:string)  [unwired: 1 in, 1 out]
                  "I: F0-ethernet 4" <- w528
                  n230 = Replace Substring(3:2 ("offset (0)"), 4:"," ("substring (\"\")"), 5:w470) -> (1:w521:string)  [unwired: 1 in, 1 out]
                  "I F0-ethernet 2" <- w521
                  n231 = Replace Substring(3:2 ("offset (0)"), 4:"," ("substring (\"\")"), 5:w487) -> (1:w519:string)  [unwired: 1 in, 1 out]
                  "I: Kamera Y" <- w519
                  n232 = Replace Substring(3:2 ("offset (0)"), 4:"," ("substring (\"\")"), 5:w504) -> (1:w516:string)  [unwired: 1 in, 1 out]
                  "I F0-ethernet 3" <- w516
                  n233 = Replace Substring(3:2 ("offset (0)"), 4:"," ("substring (\"\")"), 5:w497) -> (1:w518:string)  [unwired: 1 in, 1 out]
                  "I: BK1" <- w518
                  n234 = Replace Substring(3:2 ("offset (0)"), 4:"," ("substring (\"\")"), 5:w454) -> (1:w526:string)  [unwired: 1 in, 1 out]
                  "I: F0-ethernet 5" <- w526
                  n235 = Replace Substring(3:2 ("offset (0)"), 4:"," ("substring (\"\")"), 5:w461) -> (1:w524:string)  [unwired: 1 in, 1 out]
                  "I F0-ethernet 1" <- w524
                  n236 = Replace Substring(3:2 ("offset (0)"), 4:"," ("substring (\"\")"), 5:w481) -> (1:w530:string)  [unwired: 1 in, 1 out]
                  "I 0_3" <- w530
                  n237 = Multiply(x=w462, y=u32 1000) -> (x*y=w464:u32)
                  n238 = Multiply(x=w510, y=u32 1000) -> (x*y=w508:u32)
                  n239 = Multiply(x=w447, y=u32 1000) -> (x*y=w445:u32)
                  n240 = Multiply(x=w485, y=u32 1000) -> (x*y=w483:u32)
                  n241 = Multiply(x=w493, y=u32 1000) -> (x*y=w491:u32)
                  n242 = Multiply(x=w458, y=u32 1000) -> (x*y=w456:u32)
                  n243 = Multiply(x=w471, y=u32 1000) -> (x*y=w473:u32)
                  n244 = Multiply(x=w501, y=u32 1000) -> (x*y=w499:u32)
                  n245 = To Long Integer(number=w464) -> (32bit integer=w460:i32)
                  n246 = To Long Integer(number=w508) -> (32bit integer=w506:i32)
                  n247 = To Long Integer(number=w445) -> (32bit integer=w442:i32)
                  n248 = To Long Integer(number=w483) -> (32bit integer=w479:i32)
                  n249 = To Long Integer(number=w491) -> (32bit integer=w489:i32)
                  n250 = To Long Integer(number=w456) -> (32bit integer=w453:i32)
                  n251 = To Long Integer(number=w473) -> (32bit integer=w469:i32)
                  n252 = To Long Integer(number=w499) -> (32bit integer=w496:i32)
                  n253 = Decimal String To Number(string=w516, offset=3) -> (number=w511:i32)  [unwired: 1 in, 1 out]
                  n254 = Decimal String To Number(string=w530, offset=3) -> (number=w477:i32)  [unwired: 1 in, 1 out]
                  n255 = Decimal String To Number(string=w521, offset=3) -> (number=w475:i32)  [unwired: 1 in, 1 out]
                  n256 = Decimal String To Number(string=w524, offset=3) -> (number=w466:i32)  [unwired: 1 in, 1 out]
                  n257 = Decimal String To Number(string=w526, offset=3) -> (number=w450:i32)  [unwired: 1 in, 1 out]
                  n258 = Decimal String To Number(string=w528, offset=3) -> (number=w448:i32)  [unwired: 1 in, 1 out]
                  n259 = Equal?(x=w460, y=1000) -> (x = y?=w459:bool)
                  n260 = Decimal String To Number(string=w519, offset=3) -> (number=w486:i32)  [unwired: 1 in, 1 out]
                  n261 = Decimal String To Number(string=w518, offset=3) -> (number=w502:i32)  [unwired: 1 in, 1 out]
                  n262 = Equal?(x=w506, y=1000) -> (x = y?=w505:bool)
                  n263 = Equal?(x=w469, y=1000) -> (x = y?=w468:bool)
                  n264 = Equal?(x=w442, y=1000) -> (x = y?=w441:bool)
                  n265 = Equal?(x=w479, y=1000) -> (x = y?=w480:bool)
                  n266 = Equal?(x=w489, y=1000) -> (x = y?=w488:bool)
                  n267 = Equal?(x=w496, y=1000) -> (x = y?=w495:bool)
                  n268 = Equal?(x=w453, y=1000) -> (x = y?=w452:bool)
                  n269 = case shown="True" w441 {
                    tunnel: w448 -> [w587 w593]
                    tunnel: w442 -> [_ w591]
                    tunnel: [w587 w590] -> w449
                    frame False {
                    }
                    frame True {
                      n270 = Divide(x=w593, y=10) -> (x/y=w589:dbl)
                      n271 = To Long Integer(number=w589) -> (32bit integer=w588:i32)
                      n272 = Add(x=w588, y=w591) -> (x+y=w590:i32)
                    }
                  }
                  n273 = case shown="True" w452 {
                    tunnel: w450 -> [w594 w600]
                    tunnel: w453 -> [_ w598]
                    tunnel: [w594 w597] -> w451
                    frame False {
                    }
                    frame True {
                      n274 = Divide(x=w600, y=10) -> (x/y=w596:dbl)
                      n275 = To Long Integer(number=w596) -> (32bit integer=w595:i32)
                      n276 = Add(x=w595, y=w598) -> (x+y=w597:i32)
                    }
                  }
                  n277 = case shown="True" w459 {
                    tunnel: w466 -> [w601 w607]
                    tunnel: w460 -> [_ w605]
                    tunnel: [w601 w604] -> w467
                    frame False {
                    }
                    frame True {
                      n278 = Divide(x=w607, y=10) -> (x/y=w603:dbl)
                      n279 = To Long Integer(number=w603) -> (32bit integer=w602:i32)
                      n280 = Add(x=w602, y=w605) -> (x+y=w604:i32)
                    }
                  }
                  n281 = case shown="True" w468 {
                    tunnel: w475 -> [w608 w614]
                    tunnel: w469 -> [_ w612]
                    tunnel: [w608 w611] -> w476
                    frame False {
                    }
                    frame True {
                      n282 = Divide(x=w614, y=10) -> (x/y=w610:dbl)
                      n283 = To Long Integer(number=w610) -> (32bit integer=w609:i32)
                      n284 = Add(x=w609, y=w612) -> (x+y=w611:i32)
                    }
                  }
                  n285 = case shown="True" w480 {
                    tunnel: w477 -> [w615 w621]
                    tunnel: w479 -> [_ w619]
                    tunnel: [w615 w618] -> w478
                    frame False {
                    }
                    frame True {
                      n286 = Divide(x=w621, y=10) -> (x/y=w617:dbl)
                      n287 = To Long Integer(number=w617) -> (32bit integer=w616:i32)
                      n288 = Add(x=w616, y=w619) -> (x+y=w618:i32)
                    }
                  }
                  n289 = case shown="True" w488 {
                    tunnel: w486 -> [w622 w628]
                    tunnel: w489 -> [_ w626]
                    tunnel: [w622 w625] -> w494
                    frame False {
                    }
                    frame True {
                      n290 = Divide(x=w628, y=10) -> (x/y=w624:dbl)
                      n291 = To Long Integer(number=w624) -> (32bit integer=w623:i32)
                      n292 = Add(x=w623, y=w626) -> (x+y=w625:i32)
                    }
                  }
                  n293 = case shown="True" w495 {
                    tunnel: w502 -> [w629 w635]
                    tunnel: w496 -> [_ w633]
                    tunnel: [w629 w632] -> w503
                    frame False {
                    }
                    frame True {
                      n294 = Divide(x=w635, y=10) -> (x/y=w631:dbl)
                      n295 = To Long Integer(number=w631) -> (32bit integer=w630:i32)
                      n296 = Add(x=w630, y=w633) -> (x+y=w632:i32)
                    }
                  }
                  n297 = case shown="True" w505 {
                    tunnel: w511 -> [w636 w642]
                    tunnel: w506 -> [_ w640]
                    tunnel: [w636 w639] -> w512
                    frame False {
                    }
                    frame True {
                      n298 = Divide(x=w642, y=10) -> (x/y=w638:dbl)
                      n299 = To Long Integer(number=w638) -> (32bit integer=w637:i32)
                      n300 = Add(x=w637, y=w640) -> (x+y=w639:i32)
                    }
                  }
                  n301 = Less?(x=1000, y=w467) -> (x < y?=→"F0-e 3":bool)
                  n302 = Less?(x=1000, y=w449) -> (x < y?=→"F0-e 4":bool)
                  n303 = Less?(x=1000, y=w476) -> (x < y?=→"F0-e 2":bool)
                  n304 = Less?(x=1000, y=w512) -> (x < y?=→"F0-e 1":bool)
                  n305 = Less?(x=1000, y=w451) -> (x < y?=→"F0-e 5":bool)
                  n306 = Less?(x=1000, y=w494) -> (x < y?=→"Kamera Y":bool)
                  n307 = Less?(x=1000, y=w478) -> (x < y?=→"0_3":bool)
                  n308 = Less?(x=1000, y=w503) -> (x < y?=→"BK1":bool)
                  n309 = local write "VISA resource name out"(w514) -> ()
                  "modul 03" <- w531
                }
              }
            }
            event Value Change {
              n310 = event-data() -> ()  [unwired: 1 in, 6 out]
              n311 = VISA Close(VISA resource name=refnum<visa-resource-name> "DG645", error in (no error)=w648) -> (error out=w647:errorcluster)
              n312 = VISA Close(VISA resource name=refnum<visa-resource-name> "Adam", error in (no error)=w644) -> (error out=w643:errorcluster)
            }
            event "Setup": Value Change {
              n313 = event-data() -> ()  [unwired: 1 in, 6 out]
              n314 = Equal?(x="Values start", y=u16 5) -> (x = y?=w655:bool)
              n315 = Equal?(x="Values start", y=u16 3) -> (x = y?=w654:bool)
              n316 = Format Into String(format string="TSRC%d", "Values start") -> (resulting string=w651:string)  [unwired: 2 in, 1 out]
              n317 = Or(x=w654, y=w655) -> (x .or. y?=w653:bool)
              n318 = case shown="True" w653 {
                tunnel: w652 -> [w663 w689]
                tunnel: w651 -> [w662 w690]
                tunnel: [w661 w684] -> w650
                tunnel: [w660 w683] -> w649
                frame False {
                  n319 = Concatenate Strings(w662, "\r\n") -> (w668:string)
                  n320 = flat-sequence {
                    tunnel: w668 -> [w675]
                    tunnel: w663 -> [w674]
                    tunnel: refnum<visa-resource-name> "DG645" ("VISA resource name") -> [w673]
                    tunnel: [w672] -> w670
                    tunnel: [w671] -> w669
                    tunnel: [w677] -> w664
                    tunnel: [w678] -> w665
                    tunnel: w670 -> [w678]
                    tunnel: w669 -> [w677]
                    frame #0 {
                      n321 = VISA Write(VISA resource name=w673, write buffer=w675, error in (no error)=w674) -> (VISA resource name out=w671:refnum<visa-resource-name>, error out=w672:errorcluster)  [unwired: 1 out]
                    }
                    frame #1 {
                      n322 = Wait (ms)(milliseconds to wait=u32 50) -> ()  [unwired: 1 out]
                    }
                  }
                  n323 = VISA Clear(VISA resource name=w664, error in (no error)=w665) -> (VISA resource name out=w660:refnum<visa-resource-name>, error out=w661:errorcluster)
                }
                frame True {
                  n324 = Concatenate Strings(w690, "\r\n") -> (w693:string)
                  n325 = flat-sequence {
                    tunnel: w693 -> [w698]
                    tunnel: w689 -> [w697]
                    tunnel: refnum<visa-resource-name> "DG645" ("VISA resource name") -> [w696]
                    tunnel: [w695] -> w680
                    tunnel: [w694] -> w679
                    tunnel: [w699] -> w682
                    tunnel: [w700] -> w681
                    tunnel: w680 -> [w699]
                    tunnel: w679 -> [w700]
                    tunnel: w682 -> [w704]
                    tunnel: w681 -> [w703]
                    tunnel: [w702] -> w688
                    tunnel: [w701] -> w686
                    tunnel: [w709] -> w687
                    tunnel: w688 -> [w709]
                    tunnel: [w708] -> w685
                    tunnel: w686 -> [w708]
                    frame #0 {
                      n326 = VISA Write(VISA resource name=w696, write buffer=w698, error in (no error)=w697) -> (VISA resource name out=w694:refnum<visa-resource-name>, error out=w695:errorcluster)  [unwired: 1 out]
                    }
                    frame #1 {
                    }
                    frame #2 {
                      n327 = Concatenate Strings("*TRG" ("string"), "\r\n") -> (w705:string)
                      n328 = VISA Write(VISA resource name=w703, write buffer=w705, error in (no error)=w704) -> (VISA resource name out=w701:refnum<visa-resource-name>, error out=w702:errorcluster)  [unwired: 1 out]
                    }
                    frame #3 {
                      n329 = Wait (ms)(milliseconds to wait=u32 50) -> ()  [unwired: 1 out]
                    }
                  }
                  n330 = VISA Clear(VISA resource name=w685, error in (no error)=w687) -> (VISA resource name out=w683:refnum<visa-resource-name>, error out=w684:errorcluster)
                }
              }
              n331 = local write "VISA resource name out"(w649) -> ()
            }
            event "F-R VISAR1": Value Change {
              w724 = u16 0 items=["T0"=0, "A"=2, "B"=3, "C"=4, "D"=5, "E"=6, "F"=7, "G"=8, "H"=9] ("Reference Channel (0:T0)")
              w728 = u16 2 items=["A"=2, "B"=3, "C"=4, "D"=5, "E"=6, "F"=7, "G"=8, "H"=9] ("Channel to Modify (2:A)")
              n332 = event-data() -> ()  [unwired: 1 in, 6 out]
              n333 = Subtract(x="Delay A (0 s)", y=ext 100.0) -> (x-y=w711:ext)
              n334 = Divide(x=w711, y=ext 1000000000.0) -> (x/y=w714:ext)
              n335 = Format Into String(format string="%.;DLAY%d,%d,%.12g" ("Set Delay Command"), w728, w724, w714) -> (resulting string=w727:string)  [unwired: 2 in, 1 out]
              n336 = Concatenate Strings(w727, "\r\n") -> (w726:string)
              n337 = flat-sequence {
                tunnel: w726 -> [w734]
                tunnel: w723 -> [w733]
                tunnel: refnum<visa-resource-name> "DG645" ("VISA resource name") -> [w732]
                tunnel: [w731] -> w718
                tunnel: [w730] -> w717
                tunnel: [w736] -> w719
                tunnel: [w737] -> w721
                tunnel: w718 -> [w737]
                tunnel: w717 -> [w736]
                frame #0 {
                  n338 = VISA Write(VISA resource name=w732, write buffer=w734, error in (no error)=w733) -> (VISA resource name out=w730:refnum<visa-resource-name>, error out=w731:errorcluster)  [unwired: 1 out]
                }
                frame #1 {
                  n339 = Wait (ms)(milliseconds to wait=u32 50) -> ()  [unwired: 1 out]
                }
              }
              n340 = VISA Clear(VISA resource name=w719, error in (no error)=w721) -> (VISA resource name out=w716:refnum<visa-resource-name>, error out=w720:errorcluster)
              n341 = local write "VISA resource name out"(w716) -> ()
            }
            event "F-R VISAR2": Value Change {
              w751 = u16 0 items=["T0"=0, "A"=2, "B"=3, "C"=4, "D"=5, "E"=6, "F"=7, "G"=8, "H"=9] ("Reference Channel (0:T0)")
              w755 = u16 3 items=["A"=2, "B"=3, "C"=4, "D"=5, "E"=6, "F"=7, "G"=8, "H"=9] ("Channel to Modify (2:A)")
              n342 = event-data() -> ()  [unwired: 1 in, 6 out]
              n343 = Subtract(x="Delay B (0 s)", y=ext 100.0) -> (x-y=w738:ext)
              n344 = Divide(x=w738, y=ext 1000000000.0) -> (x/y=w741:ext)
              n345 = Format Into String(format string="%.;DLAY%d,%d,%.12g" ("Set Delay Command"), w755, w751, w741) -> (resulting string=w754:string)  [unwired: 2 in, 1 out]
              n346 = Concatenate Strings(w754, "\r\n") -> (w753:string)
              n347 = flat-sequence {
                tunnel: w753 -> [w761]
                tunnel: w750 -> [w760]
                tunnel: refnum<visa-resource-name> "DG645" ("VISA resource name") -> [w759]
                tunnel: [w758] -> w745
                tunnel: [w757] -> w744
                tunnel: [w763] -> w746
                tunnel: [w764] -> w748
                tunnel: w745 -> [w764]
                tunnel: w744 -> [w763]
                frame #0 {
                  n348 = VISA Write(VISA resource name=w759, write buffer=w761, error in (no error)=w760) -> (VISA resource name out=w757:refnum<visa-resource-name>, error out=w758:errorcluster)  [unwired: 1 out]
                }
                frame #1 {
                  n349 = Wait (ms)(milliseconds to wait=u32 50) -> ()  [unwired: 1 out]
                }
              }
              n350 = VISA Clear(VISA resource name=w746, error in (no error)=w748) -> (VISA resource name out=w743:refnum<visa-resource-name>, error out=w747:errorcluster)
              n351 = local write "VISA resource name out"(w743) -> ()
            }
            event "FI": Value Change {
              w778 = u16 0 items=["T0"=0, "A"=2, "B"=3, "C"=4, "D"=5, "E"=6, "F"=7, "G"=8, "H"=9] ("Reference Channel (0:T0)")
              w782 = u16 4 items=["A"=2, "B"=3, "C"=4, "D"=5, "E"=6, "F"=7, "G"=8, "H"=9] ("Channel to Modify (2:A)")
              n352 = event-data() -> ()  [unwired: 1 in, 6 out]
              n353 = Subtract(x="Delay C (0 s)", y=ext 100.0) -> (x-y=w766:ext)
              n354 = Divide(x=w766, y=ext 1000000000.0) -> (x/y=w767:ext)
              n355 = Format Into String(format string="%.;DLAY%d,%d,%.12g" ("Set Delay Command"), w782, w778, w767) -> (resulting string=w781:string)  [unwired: 2 in, 1 out]
              n356 = Concatenate Strings(w781, "\r\n") -> (w780:string)
              n357 = flat-sequence {
                tunnel: w780 -> [w788]
                tunnel: w777 -> [w787]
                tunnel: refnum<visa-resource-name> "DG645" ("VISA resource name") -> [w786]
                tunnel: [w785] -> w772
                tunnel: [w784] -> w771
                tunnel: [w790] -> w773
                tunnel: [w791] -> w774
                tunnel: w772 -> [w791]
                tunnel: w771 -> [w790]
                frame #0 {
                  n358 = VISA Write(VISA resource name=w786, write buffer=w788, error in (no error)=w787) -> (VISA resource name out=w784:refnum<visa-resource-name>, error out=w785:errorcluster)  [unwired: 1 out]
                }
                frame #1 {
                  n359 = Wait (ms)(milliseconds to wait=u32 50) -> ()  [unwired: 1 out]
                }
              }
              n360 = VISA Clear(VISA resource name=w773, error in (no error)=w774) -> (VISA resource name out=w770:refnum<visa-resource-name>, error out=w775:errorcluster)
              n361 = local write "VISA resource name out"(w770) -> ()
            }
            event "GF": Value Change {
              w805 = u16 0 items=["T0"=0, "A"=2, "B"=3, "C"=4, "D"=5, "E"=6, "F"=7, "G"=8, "H"=9] ("Reference Channel (0:T0)")
              w809 = u16 5 items=["A"=2, "B"=3, "C"=4, "D"=5, "E"=6, "F"=7, "G"=8, "H"=9] ("Channel to Modify (2:A)")
              n362 = event-data() -> ()  [unwired: 1 in, 6 out]
              n363 = Subtract(x="Delay D (0 s)", y=ext 100.0) -> (x-y=w794:ext)
              n364 = Divide(x=w794, y=ext 1000000000.0) -> (x/y=w792:ext)
              n365 = Format Into String(format string="%.;DLAY%d,%d,%.12g" ("Set Delay Command"), w809, w805, w792) -> (resulting string=w808:string)  [unwired: 2 in, 1 out]
              n366 = Concatenate Strings(w808, "\r\n") -> (w807:string)
              n367 = flat-sequence {
                tunnel: w807 -> [w815]
                tunnel: w804 -> [w814]
                tunnel: refnum<visa-resource-name> "DG645" ("VISA resource name") -> [w813]
                tunnel: [w812] -> w799
                tunnel: [w811] -> w798
                tunnel: [w817] -> w800
                tunnel: [w818] -> w802
                tunnel: w799 -> [w818]
                tunnel: w798 -> [w817]
                frame #0 {
                  n368 = VISA Write(VISA resource name=w813, write buffer=w815, error in (no error)=w814) -> (VISA resource name out=w811:refnum<visa-resource-name>, error out=w812:errorcluster)  [unwired: 1 out]
                }
                frame #1 {
                  n369 = Wait (ms)(milliseconds to wait=u32 50) -> ()  [unwired: 1 out]
                }
              }
              n370 = VISA Clear(VISA resource name=w800, error in (no error)=w802) -> (VISA resource name out=w797:refnum<visa-resource-name>, error out=w801:errorcluster)
              n371 = local write "VISA resource name out"(w797) -> ()
            }
            event "Kamera Y": Value Change {
              w832 = u16 0 items=["T0"=0, "A"=2, "B"=3, "C"=4, "D"=5, "E"=6, "F"=7, "G"=8, "H"=9] ("Reference Channel (0:T0)")
              w836 = u16 6 items=["A"=2, "B"=3, "C"=4, "D"=5, "E"=6, "F"=7, "G"=8, "H"=9] ("Channel to Modify (2:A)")
              n372 = event-data() -> ()  [unwired: 1 in, 6 out]
              n373 = Subtract(x="Delay E (0 s)", y=ext 100.0) -> (x-y=w820:ext)
              n374 = Divide(x=w820, y=ext 1000000000.0) -> (x/y=w819:ext)
              n375 = Format Into String(format string="%.;DLAY%d,%d,%.12g" ("Set Delay Command"), w836, w832, w819) -> (resulting string=w835:string)  [unwired: 2 in, 1 out]
              n376 = Concatenate Strings(w835, "\r\n") -> (w834:string)
              n377 = flat-sequence {
                tunnel: w834 -> [w842]
                tunnel: w831 -> [w841]
                tunnel: refnum<visa-resource-name> "DG645" ("VISA resource name") -> [w840]
                tunnel: [w839] -> w826
                tunnel: [w838] -> w825
                tunnel: [w844] -> w827
                tunnel: [w845] -> w829
                tunnel: w826 -> [w845]
                tunnel: w825 -> [w844]
                frame #0 {
                  n378 = VISA Write(VISA resource name=w840, write buffer=w842, error in (no error)=w841) -> (VISA resource name out=w838:refnum<visa-resource-name>, error out=w839:errorcluster)  [unwired: 1 out]
                }
                frame #1 {
                  n379 = Wait (ms)(milliseconds to wait=u32 50) -> ()  [unwired: 1 out]
                }
              }
              n380 = VISA Clear(VISA resource name=w827, error in (no error)=w829) -> (VISA resource name out=w824:refnum<visa-resource-name>, error out=w828:errorcluster)
              n381 = local write "VISA resource name out"(w824) -> ()
            }
            event "BK1": Value Change {
              w859 = u16 0 items=["T0"=0, "A"=2, "B"=3, "C"=4, "D"=5, "E"=6, "F"=7, "G"=8, "H"=9] ("Reference Channel (0:T0)")
              w863 = u16 7 items=["A"=2, "B"=3, "C"=4, "D"=5, "E"=6, "F"=7, "G"=8, "H"=9] ("Channel to Modify (2:A)")
              n382 = event-data() -> ()  [unwired: 1 in, 6 out]
              n383 = Subtract(x="Delay F (0 s)", y=ext 100.0) -> (x-y=w847:ext)
              n384 = Divide(x=w847, y=ext 1000000000.0) -> (x/y=w846:ext)
              n385 = Format Into String(format string="%.;DLAY%d,%d,%.12g" ("Set Delay Command"), w863, w859, w846) -> (resulting string=w862:string)  [unwired: 2 in, 1 out]
              n386 = Concatenate Strings(w862, "\r\n") -> (w861:string)
              n387 = flat-sequence {
                tunnel: w861 -> [w869]
                tunnel: w858 -> [w868]
                tunnel: refnum<visa-resource-name> "DG645" ("VISA resource name") -> [w867]
                tunnel: [w866] -> w853
                tunnel: [w865] -> w852
                tunnel: [w871] -> w855
                tunnel: [w872] -> w856
                tunnel: w853 -> [w872]
                tunnel: w852 -> [w871]
                frame #0 {
                  n388 = VISA Write(VISA resource name=w867, write buffer=w869, error in (no error)=w868) -> (VISA resource name out=w865:refnum<visa-resource-name>, error out=w866:errorcluster)  [unwired: 1 out]
                }
                frame #1 {
                  n389 = Wait (ms)(milliseconds to wait=u32 50) -> ()  [unwired: 1 out]
                }
              }
              n390 = VISA Clear(VISA resource name=w855, error in (no error)=w856) -> (VISA resource name out=w851:refnum<visa-resource-name>, error out=w854:errorcluster)
              n391 = local write "VISA resource name out"(w851) -> ()
            }
            event "BK2": Value Change {
              w886 = u16 0 items=["T0"=0, "A"=2, "B"=3, "C"=4, "D"=5, "E"=6, "F"=7, "G"=8, "H"=9] ("Reference Channel (0:T0)")
              w890 = u16 8 items=["A"=2, "B"=3, "C"=4, "D"=5, "E"=6, "F"=7, "G"=8, "H"=9] ("Channel to Modify (2:A)")
              n392 = event-data() -> ()  [unwired: 1 in, 6 out]
              n393 = Subtract(x="Delay G (0 s)", y=ext 100.0) -> (x-y=w874:ext)
              n394 = Divide(x=w874, y=ext 1000000000.0) -> (x/y=w873:ext)
              n395 = Format Into String(format string="%.;DLAY%d,%d,%.12g" ("Set Delay Command"), w890, w886, w873) -> (resulting string=w889:string)  [unwired: 2 in, 1 out]
              n396 = Concatenate Strings(w889, "\r\n") -> (w888:string)
              n397 = flat-sequence {
                tunnel: w888 -> [w896]
                tunnel: w885 -> [w895]
                tunnel: refnum<visa-resource-name> "DG645" ("VISA resource name") -> [w894]
                tunnel: [w893] -> w880
                tunnel: [w892] -> w879
                tunnel: [w898] -> w881
                tunnel: [w899] -> w883
                tunnel: w880 -> [w899]
                tunnel: w879 -> [w898]
                frame #0 {
                  n398 = VISA Write(VISA resource name=w894, write buffer=w896, error in (no error)=w895) -> (VISA resource name out=w892:refnum<visa-resource-name>, error out=w893:errorcluster)  [unwired: 1 out]
                }
                frame #1 {
                  n399 = Wait (ms)(milliseconds to wait=u32 50) -> ()  [unwired: 1 out]
                }
              }
              n400 = VISA Clear(VISA resource name=w881, error in (no error)=w883) -> (VISA resource name out=w878:refnum<visa-resource-name>, error out=w882:errorcluster)
              n401 = local write "VISA resource name out"(w878) -> ()
            }
            event "BK3": Value Change {
              w913 = u16 0 items=["T0"=0, "A"=2, "B"=3, "C"=4, "D"=5, "E"=6, "F"=7, "G"=8, "H"=9] ("Reference Channel (0:T0)")
              w917 = u16 9 items=["A"=2, "B"=3, "C"=4, "D"=5, "E"=6, "F"=7, "G"=8, "H"=9] ("Channel to Modify (2:A)")
              n402 = event-data() -> ()  [unwired: 1 in, 6 out]
              n403 = Subtract(x="Delay H (0 s)", y=ext 100.0) -> (x-y=w901:ext)
              n404 = Divide(x=w901, y=ext 1000000000.0) -> (x/y=w900:ext)
              n405 = Format Into String(format string="%.;DLAY%d,%d,%.12g" ("Set Delay Command"), w917, w913, w900) -> (resulting string=w916:string)  [unwired: 2 in, 1 out]
              n406 = Concatenate Strings(w916, "\r\n") -> (w915:string)
              n407 = flat-sequence {
                tunnel: w915 -> [w923]
                tunnel: w912 -> [w922]
                tunnel: refnum<visa-resource-name> "DG645" ("VISA resource name") -> [w921]
                tunnel: [w920] -> w907
                tunnel: [w919] -> w906
                tunnel: [w925] -> w908
                tunnel: [w926] -> w910
                tunnel: w907 -> [w926]
                tunnel: w906 -> [w925]
                frame #0 {
                  n408 = VISA Write(VISA resource name=w921, write buffer=w923, error in (no error)=w922) -> (VISA resource name out=w919:refnum<visa-resource-name>, error out=w920:errorcluster)  [unwired: 1 out]
                }
                frame #1 {
                  n409 = Wait (ms)(milliseconds to wait=u32 50) -> ()  [unwired: 1 out]
                }
              }
              n410 = VISA Clear(VISA resource name=w908, error in (no error)=w910) -> (VISA resource name out=w905:refnum<visa-resource-name>, error out=w909:errorcluster)
              n411 = local write "VISA resource name out"(w905) -> ()
            }
            event "BZ2K1W": Value Change {
              n412 = event-data() -> ("NewVal"=w935:bool)  [unwired: 1 in]
              n413 = flat-sequence {
                tunnel: w935 -> [w940]
                tunnel: w934 -> [w939]
                tunnel: refnum<visa-resource-name> "Adam" ("VISA resource name") -> [w938]
                tunnel: [w937] -> w929
                tunnel: [w936] -> w928
                tunnel: [w956] -> w931
                tunnel: [w957] -> w932
                tunnel: w929 -> [w957]
                tunnel: w928 -> [w956]
                frame #0 {
                  n414 = case shown="True" w940 {
                    tunnel: [w944 w951] -> w936
                    tunnel: [w943 w950] -> w937
                    tunnel: w939 -> [w942 w949]
                    tunnel: w938 -> [w941 w948]
                    frame False {
                      n415 = Concatenate Strings("#041000" ("string"), "\r\n") -> (w947:string)
                      n416 = VISA Write(VISA resource name=w941, write buffer=w947, error in (no error)=w942) -> (VISA resource name out=w944:refnum<visa-resource-name>, error out=w943:errorcluster)  [unwired: 1 out]
                    }
                    frame True {
                      n417 = Concatenate Strings("#041001" ("string"), "\r\n") -> (w954:string)
                      n418 = VISA Write(VISA resource name=w948, write buffer=w954, error in (no error)=w949) -> (VISA resource name out=w951:refnum<visa-resource-name>, error out=w950:errorcluster)  [unwired: 1 out]
                    }
                  }
                }
                frame #1 {
                  n419 = Wait (ms)(milliseconds to wait=u32 50) -> ()  [unwired: 1 out]
                }
              }
              n420 = VISA Clear(VISA resource name=w931, error in (no error)=w932) -> (VISA resource name out=w927:refnum<visa-resource-name>, error out=w930:errorcluster)
              n421 = local write "VISA resource name out"(w927) -> ()
            }
            event "DZ1K2W": Value Change {
              n422 = event-data() -> ("NewVal"=w964:bool)  [unwired: 1 in]
              n423 = flat-sequence {
                tunnel: w964 -> [w969]
                tunnel: refnum<visa-resource-name> "Adam" ("VISA resource name") -> [w968]
                tunnel: w962 -> [w967]
                tunnel: [w971] -> w960
                tunnel: [w970] -> w959
                tunnel: [w987] -> w965
                tunnel: [w988] -> w966
                tunnel: w960 -> [w988]
                tunnel: w959 -> [w987]
                frame #0 {
                  n424 = case shown="True" w969 {
                    tunnel: [w975 w982] -> w971
                    tunnel: [w974 w981] -> w970
                    tunnel: w967 -> [w973 w980]
                    tunnel: w968 -> [w972 w979]
                    frame False {
                      n425 = Concatenate Strings("#041100" ("string"), "\r\n") -> (w978:string)
                      n426 = VISA Write(VISA resource name=w972, write buffer=w978, error in (no error)=w973) -> (VISA resource name out=w974:refnum<visa-resource-name>, error out=w975:errorcluster)  [unwired: 1 out]
                    }
                    frame True {
                      n427 = Concatenate Strings("#041101" ("string"), "\r\n") -> (w985:string)
                      n428 = VISA Write(VISA resource name=w979, write buffer=w985, error in (no error)=w980) -> (VISA resource name out=w981:refnum<visa-resource-name>, error out=w982:errorcluster)  [unwired: 1 out]
                    }
                  }
                }
                frame #1 {
                  n429 = Wait (ms)(milliseconds to wait=u32 50) -> ()  [unwired: 1 out]
                }
              }
              n430 = VISA Clear(VISA resource name=w965, error in (no error)=w966) -> (VISA resource name out=w958:refnum<visa-resource-name>, error out=w961:errorcluster)
              n431 = local write "VISA resource name out"(w958) -> ()
            }
            event "DZ2K2W": Value Change {
              n432 = event-data() -> ("NewVal"=w997:bool)  [unwired: 1 in]
              n433 = flat-sequence {
                tunnel: w997 -> [w1002]
                tunnel: refnum<visa-resource-name> "Adam" ("VISA resource name") -> [w1001]
                tunnel: w995 -> [w1000]
                tunnel: [w999] -> w991
                tunnel: [w998] -> w990
                tunnel: [w1018] -> w993
                tunnel: [w1019] -> w994
                tunnel: w991 -> [w1019]
                tunnel: w990 -> [w1018]
                frame #0 {
                  n434 = case shown="True" w1002 {
                    tunnel: [w1004 w1013] -> w999
                    tunnel: [w1003 w1012] -> w998
                    tunnel: w1001 -> [w1006 w1011]
                    tunnel: w1000 -> [w1005 w1010]
                    frame False {
                      n435 = Concatenate Strings("#041200" ("string"), "\r\n") -> (w1009:string)
                      n436 = VISA Write(VISA resource name=w1006, write buffer=w1009, error in (no error)=w1005) -> (VISA resource name out=w1003:refnum<visa-resource-name>, error out=w1004:errorcluster)  [unwired: 1 out]
                    }
                    frame True {
                      n437 = Concatenate Strings("#041201" ("string"), "\r\n") -> (w1016:string)
                      n438 = VISA Write(VISA resource name=w1011, write buffer=w1016, error in (no error)=w1010) -> (VISA resource name out=w1012:refnum<visa-resource-name>, error out=w1013:errorcluster)  [unwired: 1 out]
                    }
                  }
                }
                frame #1 {
                  n439 = Wait (ms)(milliseconds to wait=u32 50) -> ()  [unwired: 1 out]
                }
              }
              n440 = VISA Clear(VISA resource name=w993, error in (no error)=w994) -> (VISA resource name out=w989:refnum<visa-resource-name>, error out=w992:errorcluster)
              n441 = local write "VISA resource name out"(w989) -> ()
            }
            event "BZ1K2W": Value Change {
              n442 = event-data() -> ("NewVal"=w1028:bool)  [unwired: 1 in]
              n443 = flat-sequence {
                tunnel: w1028 -> [w1033]
                tunnel: refnum<visa-resource-name> "Adam" ("VISA resource name") -> [w1032]
                tunnel: w1026 -> [w1031]
                tunnel: [w1030] -> w1022
                tunnel: [w1029] -> w1021
                tunnel: [w1049] -> w1024
                tunnel: [w1050] -> w1025
                tunnel: w1022 -> [w1050]
                tunnel: w1021 -> [w1049]
                frame #0 {
                  n444 = case shown="True" w1033 {
                    tunnel: w1032 -> [w1037 w1044]
                    tunnel: w1031 -> [w1036 w1043]
                    tunnel: [w1035 w1041] -> w1030
                    tunnel: [w1034 w1042] -> w1029
                    frame False {
                      n445 = Concatenate Strings("#041300" ("string"), "\r\n") -> (w1040:string)
                      n446 = VISA Write(VISA resource name=w1037, write buffer=w1040, error in (no error)=w1036) -> (VISA resource name out=w1034:refnum<visa-resource-name>, error out=w1035:errorcluster)  [unwired: 1 out]
                    }
                    frame True {
                      n447 = Concatenate Strings("#041301" ("string"), "\r\n") -> (w1047:string)
                      n448 = VISA Write(VISA resource name=w1044, write buffer=w1047, error in (no error)=w1043) -> (VISA resource name out=w1042:refnum<visa-resource-name>, error out=w1041:errorcluster)  [unwired: 1 out]
                    }
                  }
                }
                frame #1 {
                  n449 = Wait (ms)(milliseconds to wait=u32 50) -> ()  [unwired: 1 out]
                }
              }
              n450 = VISA Clear(VISA resource name=w1024, error in (no error)=w1025) -> (VISA resource name out=w1020:refnum<visa-resource-name>, error out=w1023:errorcluster)
              n451 = local write "VISA resource name out"(w1020) -> ()
            }
            event "BZ2K2W": Value Change {
              n452 = event-data() -> ("NewVal"=w1059:bool)  [unwired: 1 in]
              n453 = flat-sequence {
                tunnel: w1059 -> [w1064]
                tunnel: refnum<visa-resource-name> "Adam" ("VISA resource name") -> [w1063]
                tunnel: w1057 -> [w1062]
                tunnel: [w1061] -> w1053
                tunnel: [w1060] -> w1052
                tunnel: [w1080] -> w1054
                tunnel: [w1081] -> w1056
                tunnel: w1053 -> [w1081]
                tunnel: w1052 -> [w1080]
                frame #0 {
                  n454 = case shown="True" w1064 {
                    tunnel: [w1066 w1075] -> w1061
                    tunnel: [w1065 w1074] -> w1060
                    tunnel: w1062 -> [w1068 w1073]
                    tunnel: w1063 -> [w1067 w1072]
                    frame False {
                      n455 = Concatenate Strings("#041400" ("string"), "\r\n") -> (w1071:string)
                      n456 = VISA Write(VISA resource name=w1067, write buffer=w1071, error in (no error)=w1068) -> (VISA resource name out=w1065:refnum<visa-resource-name>, error out=w1066:errorcluster)  [unwired: 1 out]
                    }
                    frame True {
                      n457 = Concatenate Strings("#041401" ("string"), "\r\n") -> (w1078:string)
                      n458 = VISA Write(VISA resource name=w1072, write buffer=w1078, error in (no error)=w1073) -> (VISA resource name out=w1074:refnum<visa-resource-name>, error out=w1075:errorcluster)  [unwired: 1 out]
                    }
                  }
                }
                frame #1 {
                  n459 = Wait (ms)(milliseconds to wait=u32 50) -> ()  [unwired: 1 out]
                }
              }
              n460 = VISA Clear(VISA resource name=w1054, error in (no error)=w1056) -> (VISA resource name out=w1051:refnum<visa-resource-name>, error out=w1055:errorcluster)
              n461 = local write "VISA resource name out"(w1051) -> ()
            }
            event "DZ1K1W": Value Change {
              n462 = event-data() -> ("NewVal"=w1090:bool)  [unwired: 1 in]
              n463 = flat-sequence {
                tunnel: w1090 -> [w1095]
                tunnel: refnum<visa-resource-name> "Adam" ("VISA resource name") -> [w1094]
                tunnel: w1088 -> [w1093]
                tunnel: [w1092] -> w1084
                tunnel: [w1091] -> w1083
                tunnel: [w1111] -> w1086
                tunnel: [w1112] -> w1087
                tunnel: w1084 -> [w1112]
                tunnel: w1083 -> [w1111]
                frame #0 {
                  n464 = case shown="True" w1095 {
                    tunnel: [w1099 w1106] -> w1092
                    tunnel: [w1098 w1105] -> w1091
                    tunnel: w1094 -> [w1097 w1103]
                    tunnel: w1093 -> [w1096 w1104]
                    frame False {
                      n465 = Concatenate Strings("#041500" ("string"), "\r\n") -> (w1102:string)
                      n466 = VISA Write(VISA resource name=w1097, write buffer=w1102, error in (no error)=w1096) -> (VISA resource name out=w1098:refnum<visa-resource-name>, error out=w1099:errorcluster)  [unwired: 1 out]
                    }
                    frame True {
                      n467 = Concatenate Strings("#041501" ("string"), "\r\n") -> (w1109:string)
                      n468 = VISA Write(VISA resource name=w1103, write buffer=w1109, error in (no error)=w1104) -> (VISA resource name out=w1105:refnum<visa-resource-name>, error out=w1106:errorcluster)  [unwired: 1 out]
                    }
                  }
                }
                frame #1 {
                  n469 = Wait (ms)(milliseconds to wait=u32 50) -> ()  [unwired: 1 out]
                }
              }
              n470 = VISA Clear(VISA resource name=w1086, error in (no error)=w1087) -> (VISA resource name out=w1082:refnum<visa-resource-name>, error out=w1085:errorcluster)
              n471 = local write "VISA resource name out"(w1082) -> ()
            }
            event "DZ2K1W": Value Change {
              n472 = event-data() -> ("NewVal"=w1121:bool)  [unwired: 1 in]
              n473 = flat-sequence {
                tunnel: w1121 -> [w1126]
                tunnel: refnum<visa-resource-name> "Adam" ("VISA resource name") -> [w1125]
                tunnel: w1119 -> [w1124]
                tunnel: [w1123] -> w1115
                tunnel: [w1122] -> w1114
                tunnel: [w1142] -> w1116
                tunnel: [w1143] -> w1118
                tunnel: w1115 -> [w1143]
                tunnel: w1114 -> [w1142]
                frame #0 {
                  n474 = case shown="True" w1126 {
                    tunnel: [w1130 w1136] -> w1123
                    tunnel: [w1129 w1137] -> w1122
                    tunnel: w1124 -> [w1128 w1135]
                    tunnel: w1125 -> [w1127 w1134]
                    frame False {
                      n475 = Concatenate Strings("#041600" ("string"), "\r\n") -> (w1133:string)
                      n476 = VISA Write(VISA resource name=w1127, write buffer=w1133, error in (no error)=w1128) -> (VISA resource name out=w1129:refnum<visa-resource-name>, error out=w1130:errorcluster)  [unwired: 1 out]
                    }
                    frame True {
                      n477 = Concatenate Strings("#041601" ("string"), "\r\n") -> (w1140:string)
                      n478 = VISA Write(VISA resource name=w1134, write buffer=w1140, error in (no error)=w1135) -> (VISA resource name out=w1137:refnum<visa-resource-name>, error out=w1136:errorcluster)  [unwired: 1 out]
                    }
                  }
                }
                frame #1 {
                  n479 = Wait (ms)(milliseconds to wait=u32 50) -> ()  [unwired: 1 out]
                }
              }
              n480 = VISA Clear(VISA resource name=w1116, error in (no error)=w1118) -> (VISA resource name out=w1113:refnum<visa-resource-name>, error out=w1117:errorcluster)
              n481 = local write "VISA resource name out"(w1113) -> ()
            }
            event "BZ1K1W": Value Change {
              n482 = event-data() -> ("NewVal"=w1152:bool)  [unwired: 1 in]
              n483 = flat-sequence {
                tunnel: w1152 -> [w1157]
                tunnel: refnum<visa-resource-name> "Adam" ("VISA resource name") -> [w1156]
                tunnel: w1150 -> [w1155]
                tunnel: [w1154] -> w1146
                tunnel: [w1153] -> w1145
                tunnel: [w1173] -> w1148
                tunnel: [w1174] -> w1149
                tunnel: w1146 -> [w1174]
                tunnel: w1145 -> [w1173]
                frame #0 {
                  n484 = case shown="True" w1157 {
                    tunnel: w1155 -> [w1161 w1165]
                    tunnel: w1156 -> [w1160 w1166]
                    tunnel: [w1159 w1168] -> w1154
                    tunnel: [w1158 w1167] -> w1153
                    frame False {
                      n485 = Concatenate Strings("#041700" ("string"), "\r\n") -> (w1164:string)
                      n486 = VISA Write(VISA resource name=w1160, write buffer=w1164, error in (no error)=w1161) -> (VISA resource name out=w1158:refnum<visa-resource-name>, error out=w1159:errorcluster)  [unwired: 1 out]
                    }
                    frame True {
                      n487 = Concatenate Strings("#041701" ("string"), "\r\n") -> (w1171:string)
                      n488 = VISA Write(VISA resource name=w1166, write buffer=w1171, error in (no error)=w1165) -> (VISA resource name out=w1167:refnum<visa-resource-name>, error out=w1168:errorcluster)  [unwired: 1 out]
                    }
                  }
                }
                frame #1 {
                  n489 = Wait (ms)(milliseconds to wait=u32 50) -> ()  [unwired: 1 out]
                }
              }
              n490 = VISA Clear(VISA resource name=w1148, error in (no error)=w1149) -> (VISA resource name out=w1144:refnum<visa-resource-name>, error out=w1147:errorcluster)
              n491 = local write "VISA resource name out"(w1144) -> ()
            }
            event "GF": Value Change {
              n492 = event-data() -> ("NewVal"=w1183:bool)  [unwired: 1 in]
              n493 = flat-sequence {
                tunnel: w1183 -> [w1188]
                tunnel: refnum<visa-resource-name> "Adam" ("VISA resource name") -> [w1187]
                tunnel: w1181 -> [w1186]
                tunnel: [w1185] -> w1177
                tunnel: [w1184] -> w1176
                tunnel: [w1204] -> w1179
                tunnel: [w1205] -> w1180
                tunnel: w1177 -> [w1205]
                tunnel: w1176 -> [w1204]
                frame #0 {
                  n494 = case shown="True" w1188 {
                    tunnel: [w1192 w1199] -> w1184
                    tunnel: [w1191 w1198] -> w1185
                    tunnel: w1186 -> [w1190 w1197]
                    tunnel: w1187 -> [w1189 w1196]
                    frame False {
                      n495 = Concatenate Strings("#051000" ("string"), "\r\n") -> (w1195:string)
                      n496 = VISA Write(VISA resource name=w1189, write buffer=w1195, error in (no error)=w1190) -> (VISA resource name out=w1192:refnum<visa-resource-name>, error out=w1191:errorcluster)  [unwired: 1 out]
                    }
                    frame True {
                      n497 = Concatenate Strings("#051001" ("string"), "\r\n") -> (w1202:string)
                      n498 = VISA Write(VISA resource name=w1196, write buffer=w1202, error in (no error)=w1197) -> (VISA resource name out=w1199:refnum<visa-resource-name>, error out=w1198:errorcluster)  [unwired: 1 out]
                    }
                  }
                }
                frame #1 {
                  n499 = Wait (ms)(milliseconds to wait=u32 50) -> ()  [unwired: 1 out]
                }
              }
              n500 = VISA Clear(VISA resource name=w1179, error in (no error)=w1180) -> (VISA resource name out=w1175:refnum<visa-resource-name>, error out=w1178:errorcluster)
              n501 = local write "VISA resource name out"(w1175) -> ()
            }
            event "Kamera Y": Value Change {
              n502 = event-data() -> ("NewVal"=w1214:bool)  [unwired: 1 in]
              n503 = flat-sequence {
                tunnel: w1214 -> [w1219]
                tunnel: w1213 -> [w1218]
                tunnel: refnum<visa-resource-name> "Adam" ("VISA resource name") -> [w1217]
                tunnel: [w1216] -> w1208
                tunnel: [w1215] -> w1207
                tunnel: [w1235] -> w1210
                tunnel: [w1236] -> w1211
                tunnel: w1208 -> [w1236]
                tunnel: w1207 -> [w1235]
                frame #0 {
                  n504 = case shown="True" w1219 {
                    tunnel: [w1223 w1230] -> w1216
                    tunnel: [w1222 w1229] -> w1215
                    tunnel: w1218 -> [w1221 w1228]
                    tunnel: w1217 -> [w1220 w1227]
                    frame False {
                      n505 = Concatenate Strings("#051100" ("string"), "\r\n") -> (w1226:string)
                      n506 = VISA Write(VISA resource name=w1220, write buffer=w1226, error in (no error)=w1221) -> (VISA resource name out=w1222:refnum<visa-resource-name>, error out=w1223:errorcluster)  [unwired: 1 out]
                    }
                    frame True {
                      n507 = Concatenate Strings("#051101" ("string"), "\r\n") -> (w1233:string)
                      n508 = VISA Write(VISA resource name=w1227, write buffer=w1233, error in (no error)=w1228) -> (VISA resource name out=w1229:refnum<visa-resource-name>, error out=w1230:errorcluster)  [unwired: 1 out]
                    }
                  }
                }
                frame #1 {
                  n509 = Wait (ms)(milliseconds to wait=u32 50) -> ()  [unwired: 1 out]
                }
              }
              n510 = VISA Clear(VISA resource name=w1210, error in (no error)=w1211) -> (VISA resource name out=w1206:refnum<visa-resource-name>, error out=w1209:errorcluster)
              n511 = local write "VISA resource name out"(w1206) -> ()
            }
            event "BK1": Value Change {
              n512 = event-data() -> ("NewVal"=w1245:bool)  [unwired: 1 in]
              n513 = flat-sequence {
                tunnel: w1245 -> [w1250]
                tunnel: refnum<visa-resource-name> "Adam" ("VISA resource name") -> [w1249]
                tunnel: w1243 -> [w1248]
                tunnel: [w1247] -> w1239
                tunnel: [w1246] -> w1238
                tunnel: [w1266] -> w1241
                tunnel: [w1267] -> w1242
                tunnel: w1239 -> [w1267]
                tunnel: w1238 -> [w1266]
                frame #0 {
                  n514 = case shown="True" w1250 {
                    tunnel: [w1252 w1261] -> w1247
                    tunnel: [w1251 w1260] -> w1246
                    tunnel: w1249 -> [w1254 w1259]
                    tunnel: w1248 -> [w1253 w1258]
                    frame False {
                      n515 = Concatenate Strings("#051200" ("string"), "\r\n") -> (w1257:string)
                      n516 = VISA Write(VISA resource name=w1254, write buffer=w1257, error in (no error)=w1253) -> (VISA resource name out=w1251:refnum<visa-resource-name>, error out=w1252:errorcluster)  [unwired: 1 out]
                    }
                    frame True {
                      n517 = Concatenate Strings("#051201" ("string"), "\r\n") -> (w1264:string)
                      n518 = VISA Write(VISA resource name=w1259, write buffer=w1264, error in (no error)=w1258) -> (VISA resource name out=w1260:refnum<visa-resource-name>, error out=w1261:errorcluster)  [unwired: 1 out]
                    }
                  }
                }
                frame #1 {
                  n519 = Wait (ms)(milliseconds to wait=u32 50) -> ()  [unwired: 1 out]
                }
              }
              n520 = VISA Clear(VISA resource name=w1241, error in (no error)=w1242) -> (VISA resource name out=w1237:refnum<visa-resource-name>, error out=w1240:errorcluster)
              n521 = local write "VISA resource name out"(w1237) -> ()
            }
            event "BK 2": Value Change {
              n522 = event-data() -> ("NewVal"=w1276:bool)  [unwired: 1 in]
              n523 = flat-sequence {
                tunnel: w1276 -> [w1281]
                tunnel: refnum<visa-resource-name> "Adam" ("VISA resource name") -> [w1280]
                tunnel: w1274 -> [w1279]
                tunnel: [w1278] -> w1270
                tunnel: [w1277] -> w1269
                tunnel: [w1297] -> w1272
                tunnel: [w1298] -> w1273
                tunnel: w1270 -> [w1298]
                tunnel: w1269 -> [w1297]
                frame #0 {
                  n524 = case shown="True" w1281 {
                    tunnel: w1280 -> [w1285 w1292]
                    tunnel: w1279 -> [w1284 w1291]
                    tunnel: [w1283 w1289] -> w1278
                    tunnel: [w1282 w1290] -> w1277
                    frame False {
                      n525 = Concatenate Strings("#051300" ("string"), "\r\n") -> (w1288:string)
                      n526 = VISA Write(VISA resource name=w1285, write buffer=w1288, error in (no error)=w1284) -> (VISA resource name out=w1282:refnum<visa-resource-name>, error out=w1283:errorcluster)  [unwired: 1 out]
                    }
                    frame True {
                      n527 = Concatenate Strings("#051301" ("string"), "\r\n") -> (w1295:string)
                      n528 = VISA Write(VISA resource name=w1292, write buffer=w1295, error in (no error)=w1291) -> (VISA resource name out=w1290:refnum<visa-resource-name>, error out=w1289:errorcluster)  [unwired: 1 out]
                    }
                  }
                }
                frame #1 {
                  n529 = Wait (ms)(milliseconds to wait=u32 50) -> ()  [unwired: 1 out]
                }
              }
              n530 = VISA Clear(VISA resource name=w1272, error in (no error)=w1273) -> (VISA resource name out=w1268:refnum<visa-resource-name>, error out=w1271:errorcluster)
              n531 = local write "VISA resource name out"(w1268) -> ()
            }
            event "BK3": Value Change {
              n532 = event-data() -> ("NewVal"=w1307:bool)  [unwired: 1 in]
              n533 = flat-sequence {
                tunnel: w1307 -> [w1312]
                tunnel: refnum<visa-resource-name> "Adam" ("VISA resource name") -> [w1311]
                tunnel: w1305 -> [w1310]
                tunnel: [w1309] -> w1301
                tunnel: [w1308] -> w1300
                tunnel: [w1328] -> w1303
                tunnel: [w1329] -> w1304
                tunnel: w1301 -> [w1329]
                tunnel: w1300 -> [w1328]
                frame #0 {
                  n534 = case shown="True" w1312 {
                    tunnel: [w1314 w1323] -> w1309
                    tunnel: [w1313 w1322] -> w1308
                    tunnel: w1310 -> [w1316 w1321]
                    tunnel: w1311 -> [w1315 w1320]
                    frame False {
                      n535 = Concatenate Strings("#051400" ("string"), "\r\n") -> (w1319:string)
                      n536 = VISA Write(VISA resource name=w1315, write buffer=w1319, error in (no error)=w1316) -> (VISA resource name out=w1313:refnum<visa-resource-name>, error out=w1314:errorcluster)  [unwired: 1 out]
                    }
                    frame True {
                      n537 = Concatenate Strings("#051401" ("string"), "\r\n") -> (w1326:string)
                      n538 = VISA Write(VISA resource name=w1320, write buffer=w1326, error in (no error)=w1321) -> (VISA resource name out=w1322:refnum<visa-resource-name>, error out=w1323:errorcluster)  [unwired: 1 out]
                    }
                  }
                }
                frame #1 {
                  n539 = Wait (ms)(milliseconds to wait=u32 50) -> ()  [unwired: 1 out]
                }
              }
              n540 = VISA Clear(VISA resource name=w1303, error in (no error)=w1304) -> (VISA resource name out=w1299:refnum<visa-resource-name>, error out=w1302:errorcluster)
              n541 = local write "VISA resource name out"(w1299) -> ()
            }
            event "F-R VISAR 4": Value Change {
              n542 = event-data() -> ("NewVal"=w1338:bool)  [unwired: 1 in]
              n543 = flat-sequence {
                tunnel: w1338 -> [w1343]
                tunnel: refnum<visa-resource-name> "Adam" ("VISA resource name") -> [w1342]
                tunnel: w1336 -> [w1341]
                tunnel: [w1340] -> w1332
                tunnel: [w1339] -> w1331
                tunnel: [w1359] -> w1334
                tunnel: [w1360] -> w1335
                tunnel: w1332 -> [w1360]
                tunnel: w1331 -> [w1359]
                frame #0 {
                  n544 = case shown="True" w1343 {
                    tunnel: [w1347 w1354] -> w1340
                    tunnel: [w1346 w1353] -> w1339
                    tunnel: w1342 -> [w1345 w1351]
                    tunnel: w1341 -> [w1344 w1352]
                    frame False {
                      n545 = Concatenate Strings("#051500" ("string"), "\r\n") -> (w1350:string)
                      n546 = VISA Write(VISA resource name=w1345, write buffer=w1350, error in (no error)=w1344) -> (VISA resource name out=w1346:refnum<visa-resource-name>, error out=w1347:errorcluster)  [unwired: 1 out]
                    }
                    frame True {
                      n547 = Concatenate Strings("#051501" ("string"), "\r\n") -> (w1357:string)
                      n548 = VISA Write(VISA resource name=w1351, write buffer=w1357, error in (no error)=w1352) -> (VISA resource name out=w1353:refnum<visa-resource-name>, error out=w1354:errorcluster)  [unwired: 1 out]
                    }
                  }
                }
                frame #1 {
                  n549 = Wait (ms)(milliseconds to wait=u32 50) -> ()  [unwired: 1 out]
                }
              }
              n550 = VISA Clear(VISA resource name=w1334, error in (no error)=w1335) -> (VISA resource name out=w1330:refnum<visa-resource-name>, error out=w1333:errorcluster)
              n551 = local write "VISA resource name out"(w1330) -> ()
            }
            event "F-R VISAR 3": Value Change {
              n552 = event-data() -> ("NewVal"=w1369:bool)  [unwired: 1 in]
              n553 = flat-sequence {
                tunnel: w1369 -> [w1374]
                tunnel: refnum<visa-resource-name> "Adam" ("VISA resource name") -> [w1373]
                tunnel: w1367 -> [w1372]
                tunnel: [w1371] -> w1363
                tunnel: [w1370] -> w1362
                tunnel: [w1390] -> w1365
                tunnel: [w1391] -> w1366
                tunnel: w1363 -> [w1391]
                tunnel: w1362 -> [w1390]
                frame #0 {
                  n554 = case shown="True" w1374 {
                    tunnel: [w1378 w1384] -> w1371
                    tunnel: [w1377 w1385] -> w1370
                    tunnel: w1372 -> [w1376 w1383]
                    tunnel: w1373 -> [w1375 w1382]
                    frame False {
                      n555 = Concatenate Strings("#051600" ("string"), "\r\n") -> (w1381:string)
                      n556 = VISA Write(VISA resource name=w1375, write buffer=w1381, error in (no error)=w1376) -> (VISA resource name out=w1377:refnum<visa-resource-name>, error out=w1378:errorcluster)  [unwired: 1 out]
                    }
                    frame True {
                      n557 = Concatenate Strings("#051601" ("string"), "\r\n") -> (w1388:string)
                      n558 = VISA Write(VISA resource name=w1382, write buffer=w1388, error in (no error)=w1383) -> (VISA resource name out=w1385:refnum<visa-resource-name>, error out=w1384:errorcluster)  [unwired: 1 out]
                    }
                  }
                }
                frame #1 {
                  n559 = Wait (ms)(milliseconds to wait=u32 50) -> ()  [unwired: 1 out]
                }
              }
              n560 = VISA Clear(VISA resource name=w1365, error in (no error)=w1366) -> (VISA resource name out=w1361:refnum<visa-resource-name>, error out=w1364:errorcluster)
              n561 = local write "VISA resource name out"(w1361) -> ()
            }
            event "FI": Value Change {
              n562 = event-data() -> ("NewVal"=w1400:bool)  [unwired: 1 in]
              n563 = flat-sequence {
                tunnel: w1400 -> [w1405]
                tunnel: w1399 -> [w1404]
                tunnel: refnum<visa-resource-name> "Adam" ("VISA resource name") -> [w1403]
                tunnel: [w1402] -> w1394
                tunnel: [w1401] -> w1393
                tunnel: [w1421] -> w1396
                tunnel: [w1422] -> w1397
                tunnel: w1394 -> [w1422]
                tunnel: w1393 -> [w1421]
                frame #0 {
                  n564 = case shown="True" w1405 {
                    tunnel: w1404 -> [w1409 w1413]
                    tunnel: w1403 -> [w1408 w1414]
                    tunnel: [w1407 w1416] -> w1402
                    tunnel: [w1406 w1415] -> w1401
                    frame False {
                      n565 = Concatenate Strings("#051700" ("string"), "\r\n") -> (w1412:string)
                      n566 = VISA Write(VISA resource name=w1408, write buffer=w1412, error in (no error)=w1409) -> (VISA resource name out=w1406:refnum<visa-resource-name>, error out=w1407:errorcluster)  [unwired: 1 out]
                    }
                    frame True {
                      n567 = Concatenate Strings("#051701" ("string"), "\r\n") -> (w1419:string)
                      n568 = VISA Write(VISA resource name=w1414, write buffer=w1419, error in (no error)=w1413) -> (VISA resource name out=w1415:refnum<visa-resource-name>, error out=w1416:errorcluster)  [unwired: 1 out]
                    }
                  }
                }
                frame #1 {
                  n569 = Wait (ms)(milliseconds to wait=u32 50) -> ()  [unwired: 1 out]
                }
              }
              n570 = VISA Clear(VISA resource name=w1396, error in (no error)=w1397) -> (VISA resource name out=w1392:refnum<visa-resource-name>, error out=w1395:errorcluster)
              n571 = local write "VISA resource name out"(w1392) -> ()
            }
            event "rele 0_6": Value Change {
              n572 = event-data() -> ("NewVal"=w1431:bool)  [unwired: 1 in]
              n573 = flat-sequence {
                tunnel: w1431 -> [w1436]
                tunnel: refnum<visa-resource-name> "Adam" ("VISA resource name") -> [w1435]
                tunnel: w1429 -> [w1434]
                tunnel: [w1433] -> w1425
                tunnel: [w1432] -> w1424
                tunnel: [w1452] -> w1427
                tunnel: [w1453] -> w1428
                tunnel: w1425 -> [w1453]
                tunnel: w1424 -> [w1452]
                frame #0 {
                  n574 = case shown="True" w1436 {
                    tunnel: [w1440 w1447] -> w1432
                    tunnel: [w1439 w1446] -> w1433
                    tunnel: w1434 -> [w1438 w1445]
                    tunnel: w1435 -> [w1437 w1444]
                    frame False {
                      n575 = Concatenate Strings("#061000" ("string"), "\r\n") -> (w1443:string)
                      n576 = VISA Write(VISA resource name=w1437, write buffer=w1443, error in (no error)=w1438) -> (VISA resource name out=w1440:refnum<visa-resource-name>, error out=w1439:errorcluster)  [unwired: 1 out]
                    }
                    frame True {
                      n577 = Concatenate Strings("#061001" ("string"), "\r\n") -> (w1450:string)
                      n578 = VISA Write(VISA resource name=w1444, write buffer=w1450, error in (no error)=w1445) -> (VISA resource name out=w1447:refnum<visa-resource-name>, error out=w1446:errorcluster)  [unwired: 1 out]
                    }
                  }
                }
                frame #1 {
                  n579 = Wait (ms)(milliseconds to wait=u32 50) -> ()  [unwired: 1 out]
                }
              }
              n580 = VISA Clear(VISA resource name=w1427, error in (no error)=w1428) -> (VISA resource name out=w1423:refnum<visa-resource-name>, error out=w1426:errorcluster)
              n581 = local write "VISA resource name out"(w1423) -> ()
            }
            event "F0-ethernet 4": Value Change {
              n582 = event-data() -> ("NewVal"=w1462:bool)  [unwired: 1 in]
              n583 = flat-sequence {
                tunnel: w1462 -> [w1467]
                tunnel: refnum<visa-resource-name> "Adam" ("VISA resource name") -> [w1466]
                tunnel: w1460 -> [w1465]
                tunnel: [w1464] -> w1456
                tunnel: [w1463] -> w1455
                tunnel: [w1483] -> w1458
                tunnel: [w1484] -> w1459
                tunnel: w1456 -> [w1484]
                tunnel: w1455 -> [w1483]
                frame #0 {
                  n584 = case shown="True" w1467 {
                    tunnel: [w1471 w1478] -> w1464
                    tunnel: [w1470 w1477] -> w1463
                    tunnel: w1465 -> [w1469 w1476]
                    tunnel: w1466 -> [w1468 w1475]
                    frame False {
                      n585 = Concatenate Strings("#061100" ("string"), "\r\n") -> (w1474:string)
                      n586 = VISA Write(VISA resource name=w1468, write buffer=w1474, error in (no error)=w1469) -> (VISA resource name out=w1470:refnum<visa-resource-name>, error out=w1471:errorcluster)  [unwired: 1 out]
                    }
                    frame True {
                      n587 = Concatenate Strings("#061101" ("string"), "\r\n") -> (w1481:string)
                      n588 = VISA Write(VISA resource name=w1475, write buffer=w1481, error in (no error)=w1476) -> (VISA resource name out=w1477:refnum<visa-resource-name>, error out=w1478:errorcluster)  [unwired: 1 out]
                    }
                  }
                }
                frame #1 {
                  n589 = Wait (ms)(milliseconds to wait=u32 50) -> ()  [unwired: 1 out]
                }
              }
              n590 = VISA Clear(VISA resource name=w1458, error in (no error)=w1459) -> (VISA resource name out=w1454:refnum<visa-resource-name>, error out=w1457:errorcluster)
              n591 = local write "VISA resource name out"(w1454) -> ()
            }
            event "F0-ethernet 5": Value Change {
              n592 = event-data() -> ("NewVal"=w1493:bool)  [unwired: 1 in]
              n593 = flat-sequence {
                tunnel: w1493 -> [w1498]
                tunnel: refnum<visa-resource-name> "Adam" ("VISA resource name") -> [w1497]
                tunnel: w1491 -> [w1496]
                tunnel: [w1495] -> w1487
                tunnel: [w1494] -> w1486
                tunnel: [w1514] -> w1489
                tunnel: [w1515] -> w1490
                tunnel: w1487 -> [w1515]
                tunnel: w1486 -> [w1514]
                frame #0 {
                  n594 = case shown="True" w1498 {
                    tunnel: [w1500 w1509] -> w1495
                    tunnel: [w1499 w1508] -> w1494
                    tunnel: w1497 -> [w1502 w1507]
                    tunnel: w1496 -> [w1501 w1506]
                    frame False {
                      n595 = Concatenate Strings("#061200" ("string"), "\r\n") -> (w1505:string)
                      n596 = VISA Write(VISA resource name=w1502, write buffer=w1505, error in (no error)=w1501) -> (VISA resource name out=w1499:refnum<visa-resource-name>, error out=w1500:errorcluster)  [unwired: 1 out]
                    }
                    frame True {
                      n597 = Concatenate Strings("#061201" ("string"), "\r\n") -> (w1512:string)
                      n598 = VISA Write(VISA resource name=w1507, write buffer=w1512, error in (no error)=w1506) -> (VISA resource name out=w1508:refnum<visa-resource-name>, error out=w1509:errorcluster)  [unwired: 1 out]
                    }
                  }
                }
                frame #1 {
                  n599 = Wait (ms)(milliseconds to wait=u32 50) -> ()  [unwired: 1 out]
                }
              }
              n600 = VISA Clear(VISA resource name=w1489, error in (no error)=w1490) -> (VISA resource name out=w1485:refnum<visa-resource-name>, error out=w1488:errorcluster)
              n601 = local write "VISA resource name out"(w1485) -> ()
            }
            event "F0-ethernet 1": Value Change {
              n602 = event-data() -> ("NewVal"=w1524:bool)  [unwired: 1 in]
              n603 = flat-sequence {
                tunnel: w1524 -> [w1529]
                tunnel: refnum<visa-resource-name> "Adam" ("VISA resource name") -> [w1528]
                tunnel: w1522 -> [w1527]
                tunnel: [w1526] -> w1518
                tunnel: [w1525] -> w1517
                tunnel: [w1545] -> w1520
                tunnel: [w1546] -> w1521
                tunnel: w1518 -> [w1546]
                tunnel: w1517 -> [w1545]
                frame #0 {
                  n604 = case shown="True" w1529 {
                    tunnel: w1528 -> [w1533 w1540]
                    tunnel: w1527 -> [w1532 w1539]
                    tunnel: [w1531 w1537] -> w1526
                    tunnel: [w1530 w1538] -> w1525
                    frame False {
                      n605 = Concatenate Strings("#061300" ("string"), "\r\n") -> (w1536:string)
                      n606 = VISA Write(VISA resource name=w1533, write buffer=w1536, error in (no error)=w1532) -> (VISA resource name out=w1530:refnum<visa-resource-name>, error out=w1531:errorcluster)  [unwired: 1 out]
                    }
                    frame True {
                      n607 = Concatenate Strings("#061301" ("string"), "\r\n") -> (w1543:string)
                      n608 = VISA Write(VISA resource name=w1540, write buffer=w1543, error in (no error)=w1539) -> (VISA resource name out=w1538:refnum<visa-resource-name>, error out=w1537:errorcluster)  [unwired: 1 out]
                    }
                  }
                }
                frame #1 {
                  n609 = Wait (ms)(milliseconds to wait=u32 50) -> ()  [unwired: 1 out]
                }
              }
              n610 = VISA Clear(VISA resource name=w1520, error in (no error)=w1521) -> (VISA resource name out=w1516:refnum<visa-resource-name>, error out=w1519:errorcluster)
              n611 = local write "VISA resource name out"(w1516) -> ()
            }
            event "F0-ethernet 2": Value Change {
              n612 = event-data() -> ("NewVal"=w1555:bool)  [unwired: 1 in]
              n613 = flat-sequence {
                tunnel: w1555 -> [w1560]
                tunnel: refnum<visa-resource-name> "Adam" ("VISA resource name") -> [w1559]
                tunnel: w1553 -> [w1558]
                tunnel: [w1557] -> w1549
                tunnel: [w1556] -> w1548
                tunnel: [w1576] -> w1551
                tunnel: [w1577] -> w1552
                tunnel: w1549 -> [w1577]
                tunnel: w1548 -> [w1576]
                frame #0 {
                  n614 = case shown="True" w1560 {
                    tunnel: [w1562 w1571] -> w1557
                    tunnel: [w1561 w1570] -> w1556
                    tunnel: w1558 -> [w1564 w1569]
                    tunnel: w1559 -> [w1563 w1568]
                    frame False {
                      n615 = Concatenate Strings("#061400" ("string"), "\r\n") -> (w1567:string)
                      n616 = VISA Write(VISA resource name=w1563, write buffer=w1567, error in (no error)=w1564) -> (VISA resource name out=w1561:refnum<visa-resource-name>, error out=w1562:errorcluster)  [unwired: 1 out]
                    }
                    frame True {
                      n617 = Concatenate Strings("#061401" ("string"), "\r\n") -> (w1574:string)
                      n618 = VISA Write(VISA resource name=w1568, write buffer=w1574, error in (no error)=w1569) -> (VISA resource name out=w1570:refnum<visa-resource-name>, error out=w1571:errorcluster)  [unwired: 1 out]
                    }
                  }
                }
                frame #1 {
                  n619 = Wait (ms)(milliseconds to wait=u32 50) -> ()  [unwired: 1 out]
                }
              }
              n620 = VISA Clear(VISA resource name=w1551, error in (no error)=w1552) -> (VISA resource name out=w1547:refnum<visa-resource-name>, error out=w1550:errorcluster)
              n621 = local write "VISA resource name out"(w1547) -> ()
            }
            event "PZS 1 DOP": Value Change {
              n622 = event-data() -> ("NewVal"=w1586:bool)  [unwired: 1 in]
              n623 = flat-sequence {
                tunnel: w1586 -> [w1591]
                tunnel: refnum<visa-resource-name> "Adam" ("VISA resource name") -> [w1590]
                tunnel: w1584 -> [w1589]
                tunnel: [w1588] -> w1580
                tunnel: [w1587] -> w1579
                tunnel: [w1607] -> w1582
                tunnel: [w1608] -> w1583
                tunnel: w1580 -> [w1608]
                tunnel: w1579 -> [w1607]
                frame #0 {
                  n624 = case shown="True" w1591 {
                    tunnel: [w1595 w1602] -> w1588
                    tunnel: [w1594 w1601] -> w1587
                    tunnel: w1590 -> [w1593 w1599]
                    tunnel: w1589 -> [w1592 w1600]
                    frame False {
                      n625 = Concatenate Strings("#061500" ("string"), "\r\n") -> (w1598:string)
                      n626 = VISA Write(VISA resource name=w1593, write buffer=w1598, error in (no error)=w1592) -> (VISA resource name out=w1594:refnum<visa-resource-name>, error out=w1595:errorcluster)  [unwired: 1 out]
                    }
                    frame True {
                      n627 = Concatenate Strings("#061501" ("string"), "\r\n") -> (w1605:string)
                      n628 = VISA Write(VISA resource name=w1599, write buffer=w1605, error in (no error)=w1600) -> (VISA resource name out=w1601:refnum<visa-resource-name>, error out=w1602:errorcluster)  [unwired: 1 out]
                    }
                  }
                }
                frame #1 {
                  n629 = Wait (ms)(milliseconds to wait=u32 50) -> ()  [unwired: 1 out]
                }
              }
              n630 = VISA Clear(VISA resource name=w1582, error in (no error)=w1583) -> (VISA resource name out=w1578:refnum<visa-resource-name>, error out=w1581:errorcluster)
              n631 = local write "VISA resource name out"(w1578) -> ()
            }
            event "PZS 2 DOP": Value Change {
              n632 = event-data() -> ("NewVal"=w1617:bool)  [unwired: 1 in]
              n633 = flat-sequence {
                tunnel: w1617 -> [w1622]
                tunnel: refnum<visa-resource-name> "Adam" ("VISA resource name") -> [w1621]
                tunnel: w1615 -> [w1620]
                tunnel: [w1619] -> w1611
                tunnel: [w1618] -> w1610
                tunnel: [w1638] -> w1613
                tunnel: [w1639] -> w1614
                tunnel: w1611 -> [w1639]
                tunnel: w1610 -> [w1638]
                frame #0 {
                  n634 = case shown="True" w1622 {
                    tunnel: [w1626 w1632] -> w1619
                    tunnel: [w1625 w1633] -> w1618
                    tunnel: w1620 -> [w1624 w1631]
                    tunnel: w1621 -> [w1623 w1630]
                    frame False {
                      n635 = Concatenate Strings("#061600" ("string"), "\r\n") -> (w1629:string)
                      n636 = VISA Write(VISA resource name=w1623, write buffer=w1629, error in (no error)=w1624) -> (VISA resource name out=w1625:refnum<visa-resource-name>, error out=w1626:errorcluster)  [unwired: 1 out]
                    }
                    frame True {
                      n637 = Concatenate Strings("#061601" ("string"), "\r\n") -> (w1636:string)
                      n638 = VISA Write(VISA resource name=w1630, write buffer=w1636, error in (no error)=w1631) -> (VISA resource name out=w1633:refnum<visa-resource-name>, error out=w1632:errorcluster)  [unwired: 1 out]
                    }
                  }
                }
                frame #1 {
                  n639 = Wait (ms)(milliseconds to wait=u32 50) -> ()  [unwired: 1 out]
                }
              }
              n640 = VISA Clear(VISA resource name=w1613, error in (no error)=w1614) -> (VISA resource name out=w1609:refnum<visa-resource-name>, error out=w1612:errorcluster)
              n641 = local write "VISA resource name out"(w1609) -> ()
            }
            event "F0-ethernet 3": Value Change {
              n642 = event-data() -> ("NewVal"=w1648:bool)  [unwired: 1 in]
              n643 = flat-sequence {
                tunnel: w1648 -> [w1653]
                tunnel: refnum<visa-resource-name> "Adam" ("VISA resource name") -> [w1652]
                tunnel: w1646 -> [w1651]
                tunnel: [w1650] -> w1642
                tunnel: [w1649] -> w1641
                tunnel: [w1669] -> w1644
                tunnel: [w1670] -> w1645
                tunnel: w1642 -> [w1670]
                tunnel: w1641 -> [w1669]
                frame #0 {
                  n644 = case shown="True" w1653 {
                    tunnel: w1651 -> [w1657 w1661]
                    tunnel: w1652 -> [w1656 w1662]
                    tunnel: [w1655 w1664] -> w1650
                    tunnel: [w1654 w1663] -> w1649
                    frame False {
                      n645 = Concatenate Strings("#061700" ("string"), "\r\n") -> (w1660:string)
                      n646 = VISA Write(VISA resource name=w1656, write buffer=w1660, error in (no error)=w1657) -> (VISA resource name out=w1654:refnum<visa-resource-name>, error out=w1655:errorcluster)  [unwired: 1 out]
                    }
                    frame True {
                      n647 = Concatenate Strings("#061701" ("string"), "\r\n") -> (w1667:string)
                      n648 = VISA Write(VISA resource name=w1662, write buffer=w1667, error in (no error)=w1661) -> (VISA resource name out=w1663:refnum<visa-resource-name>, error out=w1664:errorcluster)  [unwired: 1 out]
                    }
                  }
                }
                frame #1 {
                  n649 = Wait (ms)(milliseconds to wait=u32 50) -> ()  [unwired: 1 out]
                }
              }
              n650 = VISA Clear(VISA resource name=w1644, error in (no error)=w1645) -> (VISA resource name out=w1640:refnum<visa-resource-name>, error out=w1643:errorcluster)
              n651 = local write "VISA resource name out"(w1640) -> ()
            }
          }
          "error out" <- w12
          "error out 2" <- w11
          n652 = Get Date/Time In Seconds() -> (seconds since 1Jan1904=→"Time Stamp":timestamp)
          n653 = VISA Close(VISA resource name=w17, error in (no error)=w12) -> (error out=w18:errorcluster)
          n654 = VISA Close(VISA resource name=w16, error in (no error)=w15) -> ()  [unwired: 1 out]
          n655 = VISA Close(VISA resource name=w13, error in (no error)=w14) -> ()  [unwired: 1 out]
        }
      }
    }
  }
  n656 = invoke class="IWebBrowser2" method="Navigate2"(reference="WebBrowser", "URL"="http://192.168.1.42/") -> ()  [unwired: 6 in, 8 out]
